vi "Measurement.vi"(0 "Position":T7(array[cluster]) {"Z" format="%.1f"; "Y" format="%.1f"; "X" format="%.1f"}, 1 "setup":T8=enum."Show Setup", 2 "Post Process":T5, 4 "File":T9, 5 "Results file":path, 7 "Raw data file":path, 11 "Setup filename":string) -> (14 "2nd plot":cluster{"Xo":dbl, "Delta X":dbl, dbl[]}[](graph), 19 "Status Out":T4)   [LabVIEW 2011]
uses:
  Anemometry Sub Vis/Controls/Save_Data.ctl
  Anemometry Sub Vis/Controls/Setup.ctl
  Anemometry Sub Vis/Controls/Graph_Type.ctl
  Anemometry Sub Vis/Controls/Post_Process.ctl
  Anemometry Sub Vis/Gen Trav/Multi_Run_Status.ctl
  Anemometry Sub Vis/Controls/Board_Types.ctl
  Anemometry Sub Vis/File/Setup_Filetype.ctl
  Anemometry Sub Vis/Controls/Block_start_and_end.ctl
  ADAM Client/Sub VIs/ADAM Controls/Traverse_Level_State.ctl
  Anemometry Sub Vis/Globals/Trav_pos_global.vi
  Anemometry Sub Vis/Globals/Meas_global.vi
  Anemometry Sub Vis/Acquisition/Data_Translation/DataTranslation_global.vi
  Anemometry Sub Vis/Acquisition/PWA/PWAtasksGLOBAL.vi
  Anemometry Sub Vis/Globals/Preference_global.vi
  Anemometry Sub Vis/Globals/LDA_meas_global_2.vi
  Anemometry Sub Vis/Globals/LDA_meas_global_1.vi
  Anemometry Sub Vis/Globals/Dynamic_call_global.ph.vi
  Anemometry Sub Vis/Globals/Plug_in_data_global.vi
panel:
  in  "PP next block":bool
  out "Pause message":string
  out "Statistics":string[][](table)
  in  "Tab Control":T1(tab)
  out "Measurement time (min)":dbl=6.0 format="%.2f"
  in  "No of bins":i32=80
  in  "Show Smoth":bool=TRUE
  in  "Second Graph":T3={"Plot 1"=2, "Plot 2"=1, "Save graph"=0, "Plot Type"=enum."Vel histogram"} {"Save graph" items=["Do not save plot", "Save plot"]; "Plot 2" items=["Nothing", "LDA (U1)", "LDA (U2)", "HW (Uhw) LDA Sync", "HW (Uhw)", "RV (Sync)"]; "Plot 1" items=["Nothing", "LDA (U1)", "LDA (U2)", "HW (Uhw) LDA Sync", "HW (Uhw)", "RV (Sync)"]}
  in  "First Graph":T3={"Plot 1"=1, "Plot 2"=2, "Save graph"=0, "Plot Type"=enum."Velocity trace"} {"Save graph" items=["Do not save plot", "Save plot"]; "Plot 2" items=["Nothing", "LDA (U1)", "LDA (U2)", "HW (Uhw) LDA Sync", "HW (Uhw)", "RV (Sync)"]; "Plot 1" items=["Nothing", "LDA (U1)", "LDA (U2)", "HW (Uhw) LDA Sync", "HW (Uhw)", "RV (Sync)"]}
  out "First plot":cluster{"Xo":dbl, "Delta X":dbl, dbl[]}[](graph)
  in  "Comments":string
  out "BSA Diagnostic info":string[][](table)
  out "uv":dbl[][](graph)=[[-0.041806189081711534, -0.046435429052714985, -0.04035660097427599, -0.042187605126076694, -0.042052555599004206]]
  out "u^4":dbl[][](graph)
  out "u^3":dbl[][](graph)
  out "u^2":dbl[][](graph)=[[0.09743628875280319, 0.10575821456272283, 0.10126262927293661, 0.09890442087602569, 0.1022948212436432]]
  out "U":dbl[][](graph)=[[0.8295029456391334, 0.8915896983798417, 0.8415763502225625, 0.8394746126219594, 0.8466062785395404]]
  in  "Block average display control":cluster{"Name":string, "Include":bool}[](array[cluster])=[{"Name"="FF (C)", "Include"=FALSE}]
  out "Array U":dbl[][](array[numeric]) format="%.2e"
  out "Array u^2":dbl[][](array[numeric]) format="%.2e"
  out "Actual Sampling freq":dbl=100.0 format="%.1f"
  in  "Desired Sampling freq (Hz)":dbl=100.0 format="%.1f"
  in  "Correlate?":T6(ring)
  out "Current Block No":i32=5
  in  "Pause":bool
  in  "No of Blocks":i32=5
  in  "stop":bool
  in  "No of samples":i32=1000 min=0 step=1
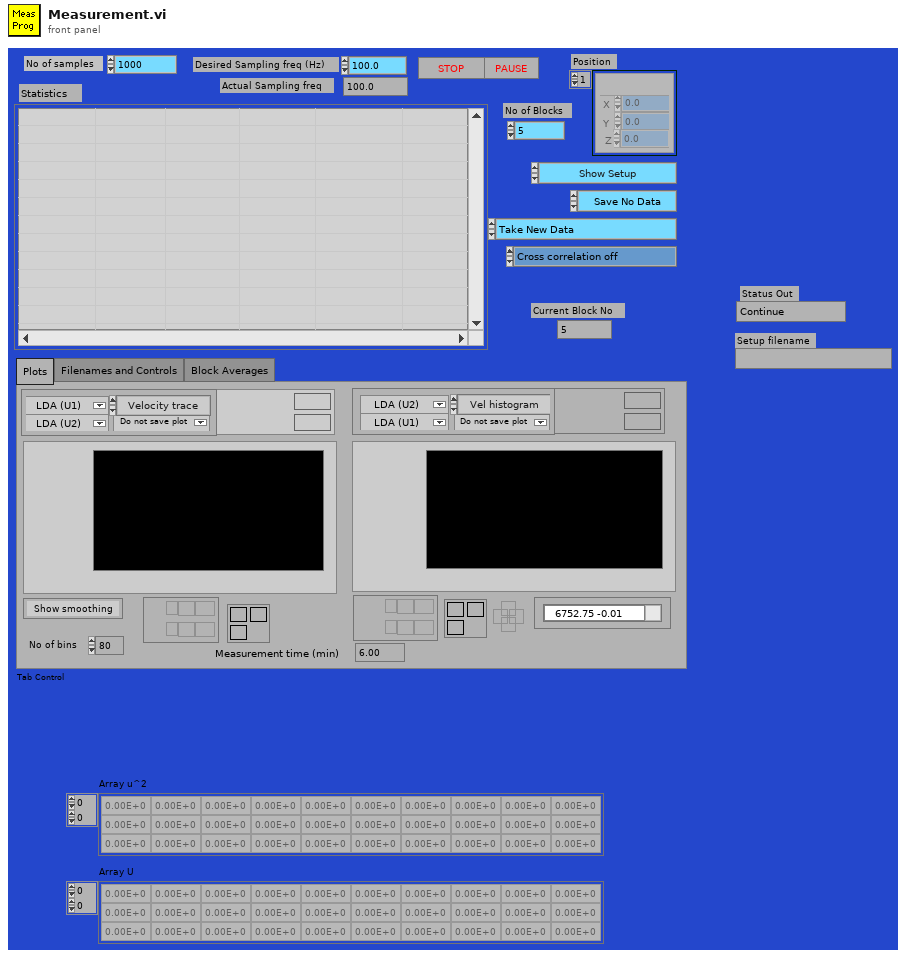
[diagram p1: front panel]
types:
  T1 = enum32{"Plots", "Filenames and Controls", "Block Averages"}
  T2 = typedef "Graph_Type.ctl" = enum16{"Show no graph", "Voltage trace", "Velocity trace", "Vel histogram", "Spectrum", "f.E(f) v Log f", "Auto-Corr"}
  T3 = cluster{"Plot 1":u16, "Plot 2":u16, "Save graph":u16, "Plot Type":T2}
  T4 = typedef "Multi_Run_Status.ctl" = enum16{"Continue", "Jump to Next Point", "Jump to Next Row", "Jump To Fall Back", "Terminate Run"}
  T5 = typedef "Post_Process.ctl" = enum16{"Take New Data", "Post Process Raw Data File"}
  T6 = enum16{"Cross correlation off", "Show correlation panel", "Correlate without activating panel"}
  T7 = cluster{"Name":string, "X":dbl, "Y":dbl, "Z":dbl}[]
  T8 = typedef "Setup.ctl" = enum16{"Run Program", "Show Setup", "Save Current Setup", "Setup Front Panel"}
  T9 = typedef "Save_Data.ctl" = enum16{"Save No Data", "Save Data"}
  T10 = enum32{"Bad", "Idle", "Run top level", "Running"}
  T11 = enum16{"Velocity", "Transit time", "Arrival time"}
  T12 = enum16{"Save no data", "Save data in new files", "Save data in existing files"}
  T13 = typedef "Board_Types.ctl" = enum16{"Simulate", "Local ADAM", "Server ADAM", "NI-DAQmx", "NI-DAQmxBase", "ADC488", "DT LV-link"}
  T14 = typedef "Setup_Filetype.ctl" = enum16{"Measurement Setups", "Calibration Setups", "General", "Results File Plotter Setups", "Speed Calib Tweaks"}
  T15 = typedef "Block_start_and_end.ctl" = cluster{"Started":dbl, "Ended":dbl, "Analogue Frequency Hz":dbl}
  T16 = typedef "Traverse_Level_State.ctl" = enum16{"Running", "Complete"}
  T17 = typedef "Traverse_cluster.ctl" = cluster{"Start X":dbl, "Start Y":dbl, "Start Z":dbl, "End X":dbl, "End Y":dbl, "End Z":dbl, "No. of pts.":i32, "Spacing":T18, "Filename":path, "Tunnel Speed":dbl, "Averaging time (min)":dbl, "Extra Commands":string, "Specific Arguments":string, "Emission Rate (l/min)":dbl, "Trace Gas Concentration (%)":dbl, "Density Ratio":string, "Comments":string, "Row No":i32, "Row Type Selector":T19, "Completion time":string, "Row Duration (mins)":dbl, "No. of Valid pts.":i32, "Meas Setup File":string}
  T18 = typedef "Spacing.ctl" = enum16{"Linear", "Log", "Gauss", "Specified", "N/A"}
  T19 = typedef "Multi_run_mode.ctl" = enum16{"Move Traverse Only", "Set Tunnel Speed Only", "Set Source Only", "Set Measurement Conditions", "Single Measurement", "Vertical Profile", "Lateral Profile", "Longitudinal Profile", "Explore Volume", "Multi-Axis Profile", "Auto Calibrate", "Meas Fast FID Bkgnd", "Check Beam Power", "Scanning Valve Measurement", "Run VI Named:", "Set ADAM Ch", "Wait (minutes)", "Send Message", "Synchronize With:", "Fall Back to this Row", "Turn Off Row Repeating", "Blank Row", "Traverse 3D Volume"}
  T20 = typedef "Analysis_info_cluster.ctl" = cluster{"Colour":u32, "Inst type":T21, "Inst name":string, "Symbol":string, "Code name":string, "Extra Info":string, "Inst Array":T22, "Index":i32, "Voltage Index":i32, "Extra Titles":string[], "Extra Values":string[], "Eng Values":dbl[], "Time (ms)":dbl[], "TT / Voltage":dbl[], "u^2":dbl, "U":dbl, "u^3/(u^2)^(1.5)":dbl, "u^4":dbl, "u^4/(u^2)^2 -3":dbl, "Mean % Err":dbl, "% u'/U":dbl}
  T21 = typedef "Inst_type.ctl" = enum16{"Propeller anemometer", "Raw voltage", "Pressure Transducer", "Pitot-static tube", "Preston tube", "Hot wire", "Cross wire 1", "Cross wire 2", "Generic Linear", "Generic Polynomial", "Generic BackPoly", "Fast FID", "Thermocouple", "Cold wire", "Pulsed Wire", "LDA Vel", "LDA Tran time", "LDA Arr time"}
  T22 = typedef "Instrument_Array.ctl" = enum16{"PWA", "LDA", "Analogue"}
  T23 = enum16{"Velocity", "Transit time", "Arrival time"}[]
  T24 = typedef "BSA_Type.ctl" = enum16{"57N11", "BSA F60"}
  T25 = typedef "BSA_info_Cluster.ctl" = cluster{"GPIB Address":string, "No of Check Bytes":i32, "Extra Info":string, "COLOUR":u32, "Wavelength (nm)":dbl}
  T26 = typedef "Ch_and_Spans.ctl" = cluster{"high limit (10V)":sgl, "low limit (-10V)":sgl, "Ch No":i16, "Var name":string, "Use Latest Calib":bool}
  T27 = typedef "Velocity_cluster.ctl" = cluster{"Name":string, "U":dbl, "u^2":dbl, "u^3/(u^2)^(1.5)":dbl, "u^4/(u^2)^2 -3":dbl, "% u'/U":dbl, "Mean % Err":dbl, "u^4":dbl}
  T28 = typedef "Analysis_type_cluster.ctl" = cluster{"Analysis type":T29, "Indicies":i32[], "Name":string, "Inst Array":T22, "Info index":i32}
  T29 = typedef "Analysis_type_Enum.ctl" = enum16{"Slow Response", "Fast Response", "Weighted Fast Response", "Fast FID", "Weighted Fast FID", "Cross Wire", "Weighted Cross Wire", "Weighted LDA"}
  T30 = cluster{"Insts for plotting[0]":u16, "Insts for plotting[1]":u16}
  T31 = typedef "PWA_Data.ctl" = enum16{"No PWA Data", "One Ch PWA"}
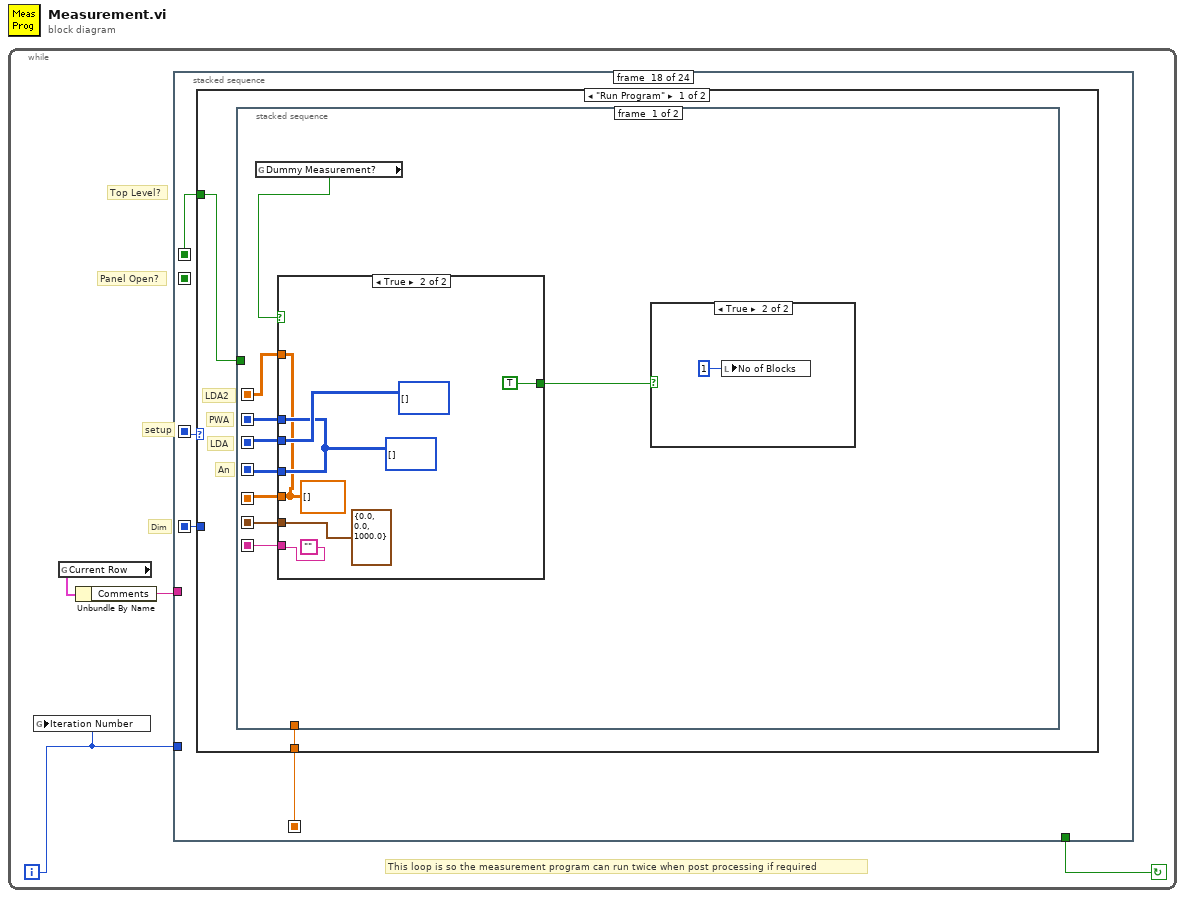
[diagram p0: block diagram]
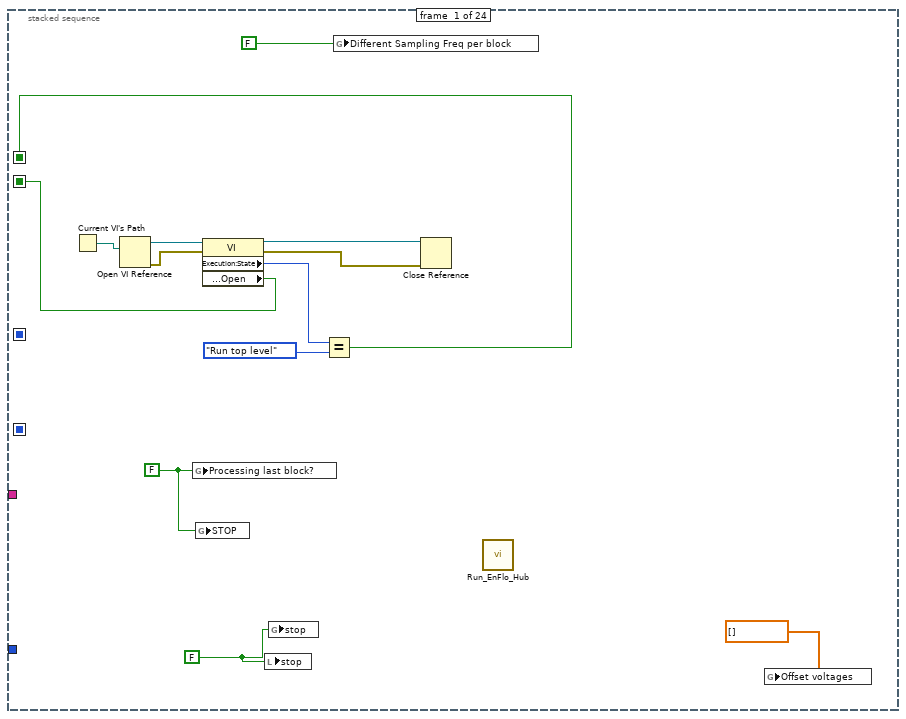
[diagram p2: hidden frame]
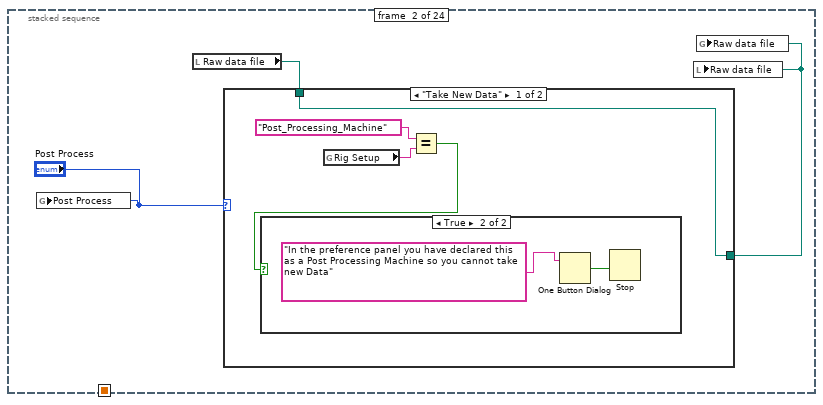
[diagram p3: hidden frame]
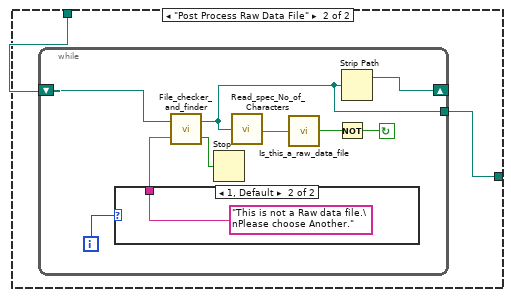
[diagram p5: hidden frame]
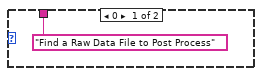
[diagram p6: hidden frame]
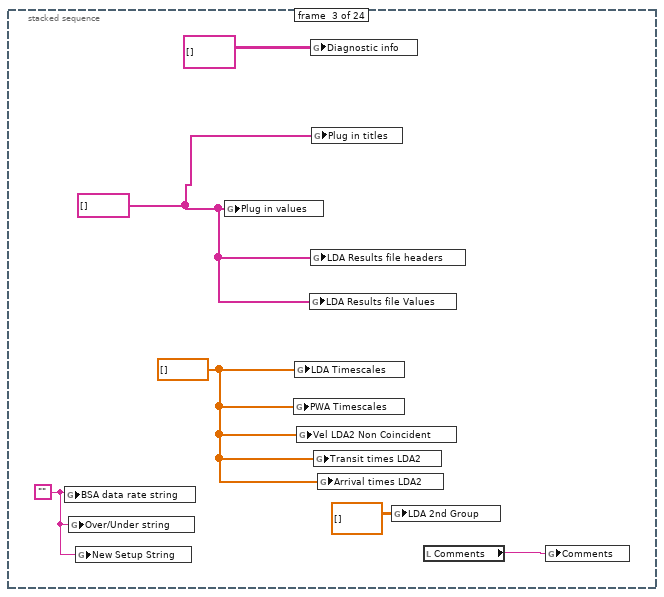
[diagram p7: hidden frame]
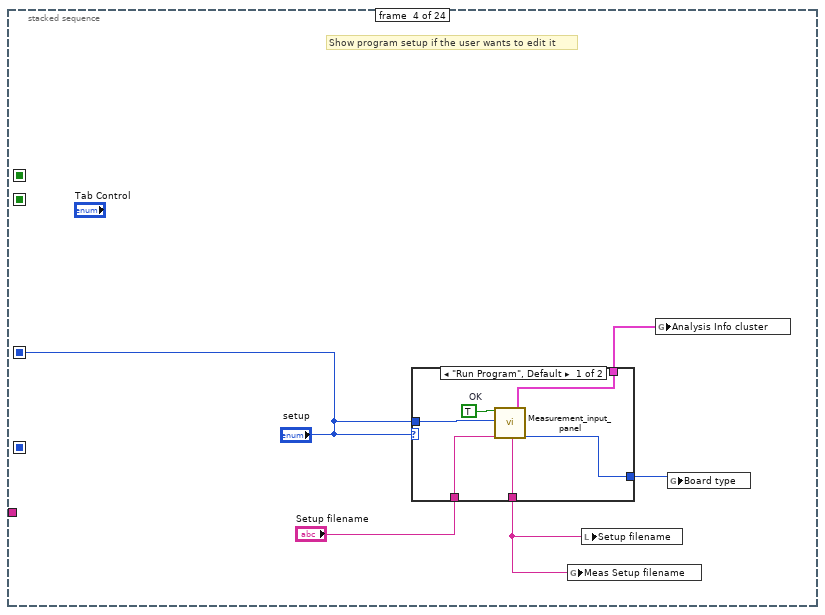
[diagram p8: hidden frame]
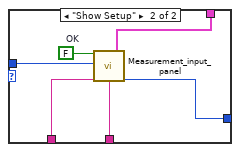
[diagram p9: hidden frame]
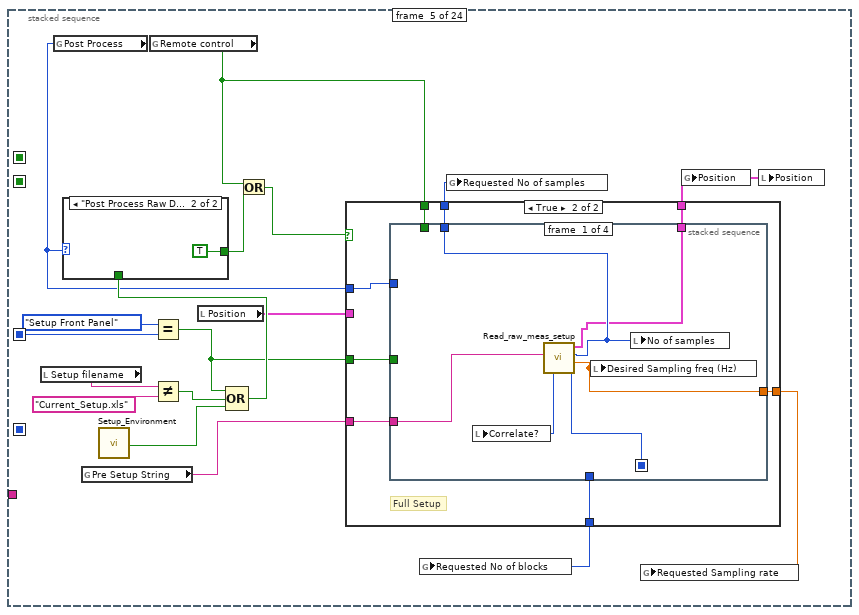
[diagram p10: hidden frame]
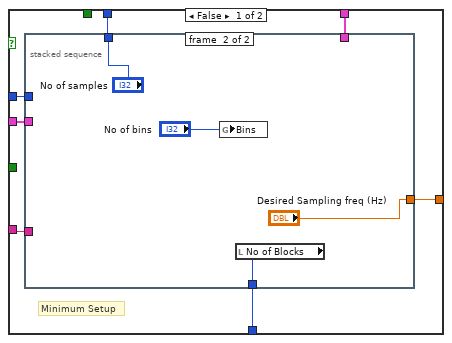
[diagram p12: hidden frame]
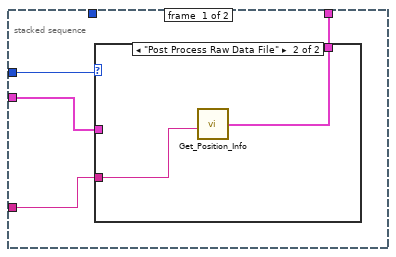
[diagram p13: hidden frame]
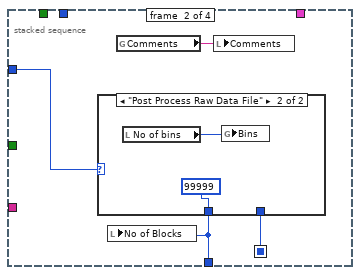
[diagram p15: hidden frame]
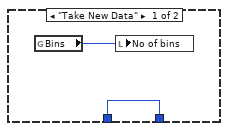
[diagram p16: hidden frame]
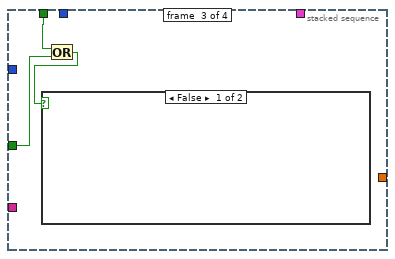
[diagram p17: hidden frame]
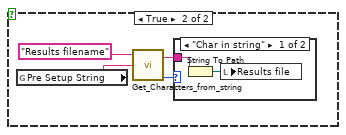
[diagram p18: hidden frame]
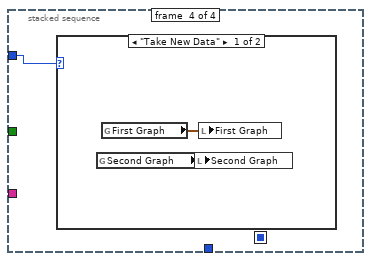
[diagram p20: hidden frame]
diagram:
  n1 = while {
    i -> [w1]
    stop <- w2 continue-if-true
    # "This loop is so the measurement program can run twice when post processing if required"
    # "Panel Open?"
    # "Top Level?"
    # "setup"
    # "Dim"
    n2 = global write "Meas_global.vi" "Iteration Number"(w1) -> ()
    n3 = global read "Trav_pos_global.vi" "Current Row"() -> (w3:T17)
    n4 = Unbundle By Name(w3) -> ("Comments"=w4:string)
    n5 = stacked-sequence {
      seq-local: [_ _ _ _ _ _ _ _ w188 _ _ _ _ _ _ _ _ _ _ _ _ _ _ _] -> [_ _ _ _ _ _ _ _ _ _ _ _ _ _ _ _ _ w627 _ _ _ _ _ _]
      seq-local: [_ _ _ "setup" _ _ _ _ _ _ _ _ _ _ _ _ _ _ _ _ _ _ _ _] -> [_ _ _ _ w72 _ _ _ w180 w265 _ _ _ _ w525 w565 w572 w628 w944 w1020 w1046 _ _ w1121]
      seq-local: [_ _ _ _ _ _ _ _ _ _ _ _ _ _ _ _ w568 _ _ _ _ _ _ _] -> [_ _ _ _ _ _ _ _ _ _ _ _ _ _ _ _ _ w626 w927 _ _ _ _ _]
      seq-local: [w7 _ _ _ _ _ _ _ _ _ _ _ _ _ _ _ _ _ _ _ _ _ _ _] -> [_ _ _ _ _ _ _ _ _ w245 _ _ _ _ w521 _ _ w625 _ _ _ _ _ _]
      seq-local: [w6 _ _ _ _ _ _ _ _ _ _ _ _ _ _ _ _ _ _ _ _ _ _ _] -> [_ _ _ _ _ _ _ _ _ _ _ _ w364 _ _ _ _ _ _ _ _ _ _ _]
      tunnel: w4 -> [_ _ _ _ _ _ _ w173 _ _ _ _ _ _ _ _ _ _ _ _ _ _ w1089 _]
      tunnel: w1 -> [_ _ _ _ _ _ _ _ _ _ _ _ _ _ _ _ _ _ _ _ _ _ w1084 _]
      tunnel: [_ _ _ _ _ _ _ _ _ _ _ _ _ _ _ _ _ _ _ _ _ _ w1083 _] -> w2
      frame #0 {
        w15 = FALSE ("Processing last block?")
        w16 = FALSE ("stop")
        n6 = Current VI's Path() -> (path=w8:path)
        n7 = Open VI Reference(vi path=w8) -> (vi reference=w9:refnum<vi>, error out=w10:errorcluster)  [unwired: 1 in, 4 out]
        n8 = global write "Meas_global.vi" "Processing last block?"(w15) -> ()
        n9 = global write "PWAtasksGLOBAL.vi" "STOP"(w15) -> ()
        n10 = property class="VI"(reference=w9, error in=w10) -> (reference out=w11:refnum<vi>, error out=w12:errorcluster, "Execution:State"=w13:T10, "Front Panel.Open"=w6:bool)
        n11 = local write "stop"(w16) -> ()
        n12 = global write "Meas_global.vi" "stop"(w16) -> ()
        n13 = Equal?(x=w13, y=T10."Run top level" ("Exec.State")) -> (x = y?=w7:bool)
        n14 = global write "DataTranslation_global.vi" "Different Sampling Freq per block"(FALSE ("Different Sampling Freq per block")) -> ()
        n15 = Close Reference(reference=w11, error in (no error)=w12) -> ()  [unwired: 1 out]
        n16 = call "Run_EnFlo_Hub.vi"() -> ()  [unwired: 8 out]
        n17 = global write "Meas_global.vi" "Offset voltages"(dbl[] [] ("Offset voltages used")) -> ()
      }
      frame #1 {
        n18 = global write "Meas_global.vi" "Post Process"("Post Process") -> ()
        n19 = local read "Raw data file"() -> (w20:path)
        n20 = case shown="\"Take New Data\"" "Post Process" {
          tunnel: [w24 w28] -> w19
          tunnel: w20 -> [w24 w27]
          frame "Take New Data" {
            n21 = global read "Preference_global.vi" "Rig Setup"() -> (w23:string)
            n22 = Equal?(x="Post_Processing_Machine" ("Rig Setup"), y=w23) -> (x = y?=w21:bool)
            n23 = case shown="True" w21 {
              frame False {
              }
              frame True {
                n24 = One Button Dialog(message="In the preference panel you have declared this as a Post Processing Machine so you cannot take new Data") -> (true=w25:bool)  [unwired: 1 in]
                n25 = Stop(stop? (T)=w25) -> ()
              }
            }
          }
          frame "Post Process Raw Data File" {
            n26 = while {
              tunnel: [w30] -> w28
              shift-left: w27 -> [w32]
              shift-right: [w31] -> _
              i -> [w33]
              stop <- w34 continue-if-true
              n27 = case shown="1, Default" w33 {
                tunnel: ["Find a Raw Data File to Post Process" ("Promp if not found") "This is not a Raw data file.\nPlease choose Another." ("Promp if not found")] -> w37
                frame 0 {
                }
                frame 1, Default {
                }
              }
              n28 = call "File_checker_and_finder.vi"("Promp if not found"=w37, "Filename In"=w32) -> ("cancelled"=w29:bool, "Filename Out"=w30:path)
              n29 = Stop(stop? (T)=w29) -> ()
              n30 = call "Read_spec_No_of_Characters.vi"("Filename"=w30) -> ("character string"=w36:string)  [unwired: 1 out]
              n31 = call "Is_this_a_raw_data_file.vi"("character string"=w36) -> ("Raw Dat File?"=w35:bool)  [unwired: 2 out]
              n32 = Not(x=w35) -> (.not. x?=w34:bool)
              n33 = Strip Path(path=w30) -> (stripped path=w31:path)  [unwired: 1 out]
            }
          }
        }
        n34 = local write "Raw data file"(w19) -> ()
        n35 = global write "Meas_global.vi" "Raw data file"(w19) -> ()
      }
      frame #2 {
        w40 = dbl[] [] ("LDA Timescales")
        w43 = string[] [] ("Plug in values")
        w45 = ""
        n36 = global write "Meas_global.vi" "BSA data rate string"(w45) -> ()
        n37 = global write "Meas_global.vi" "Over/Under string"(w45) -> ()
        n38 = global write "Meas_global.vi" "New Setup String"(w45) -> ()
        n39 = global write "Dynamic_call_global.ph.vi" "Plug in values"(w43) -> ()
        n40 = global write "PWAtasksGLOBAL.vi" "PWA Timescales"(w40) -> ()
        n41 = global write "LDA_meas_global_1.vi" "LDA Timescales"(w40) -> ()
        n42 = global write "LDA_meas_global_2.vi" "Vel LDA2 Non Coincident"(w40) -> ()
        n43 = global write "LDA_meas_global_1.vi" "LDA Results file Values"(w43) -> ()
        n44 = global write "Meas_global.vi" "Diagnostic info"(string[][] [] ("Diagnostic info")) -> ()
        n45 = global write "LDA_meas_global_1.vi" "LDA Results file headers"(w43) -> ()
        n46 = global write "Dynamic_call_global.ph.vi" "Plug in titles"(w43) -> ()
        n47 = global write "LDA_meas_global_2.vi" "Transit times LDA2"(w40) -> ()
        n48 = global write "LDA_meas_global_2.vi" "Arrival times LDA2"(w40) -> ()
        n49 = global write "LDA_meas_global_2.vi" "LDA 2nd Group"(dbl[][] [] ("LDA 2nd Group")) -> ()
        n50 = local read "Comments"() -> (w44:string)
        n51 = global write "Meas_global.vi" "Comments"(w44) -> ()
      }
      frame #3 {
        # "Show program setup if the user wants to edit it"
        n52 = case shown="\"Run Program\", Default" "setup" {
          tunnel: [w55 w61] -> w50
          tunnel: [w54 w60] -> w49
          tunnel: "Setup filename" -> [w53 w59]
          tunnel: [w52 w58] -> w46
          tunnel: "setup" -> [w51 w57]
          frame "Run Program", Default {
            w56 = TRUE  # OK
            n53 = call "Measurement_input_panel.vi"("OK"=w56, "setup"=w51, "Setup filename"=w53) -> ("Setup filename out"=w52:string, "Analysis Info cluster"=w55:T20[], "Board type"=w54:T13)  [unwired: 14 out]
          }
          frame "Show Setup" {
            w62 = FALSE  # OK
            n54 = call "Measurement_input_panel.vi"("OK"=w62, "setup"=w57, "Setup filename"=w59) -> ("Setup filename out"=w58:string, "Analysis Info cluster"=w61:T20[], "Board type"=w60:T13)  [unwired: 14 out]
          }
        }
        n55 = global write "Meas_global.vi" "Meas Setup filename"(w46) -> ()
        n56 = local write "Setup filename"(w46) -> ()
        n57 = global write "Meas_global.vi" "Analysis Info cluster"(w50) -> ()
        n58 = global write "Meas_global.vi" "Board type"(w49) -> ()
      }
      frame #4 {
        n59 = local read "Setup filename"() -> (w76:string)
        n60 = global read "Meas_global.vi" "Post Process"() -> (w71:T5)
        n61 = global read "Meas_global.vi" "Pre Setup String"() -> (w67:string)
        n62 = call "Setup_Environment.vi"() -> ("First Time"=w68:bool)  [unwired: 1 in]
        n63 = global read "Meas_global.vi" "Remote control"() -> (w64:bool)
        n64 = Equal?(x=Setup."Setup Front Panel" ("setup"), y=w72) -> (x = y?=w63:bool)
        n65 = Not Equal?(x=w76, y="Current_Setup.xls" ("Setup filename")) -> (x != y?=w74:bool)
        n66 = local read "Position"() -> (w65:T7)
        n67 = Compound Arithmetic op=OR(w63, w74, w68) -> (w73:bool)
        n68 = case shown="\"Post Process Raw Data File\"" w71 {
          tunnel: [w81 TRUE] -> w80
          tunnel: w73 -> [w81 _]
          frame "Take New Data" {
          }
          frame "Post Process Raw Data File" {
          }
        }
        n69 = Or(x=w64, y=w80) -> (x .or. y?=w79:bool)
        n70 = case shown="True" w79 {
          tunnel: w71 -> [w85 w108]
          tunnel: [w89 w107] -> w69
          tunnel: [w88 w102] -> w78
          tunnel: [w87 w106] -> w77
          tunnel: [w86 w105] -> w66
          tunnel: w67 -> [w84 w104]
          tunnel: w65 -> [w83 _]
          tunnel: w64 -> [_ w103]
          tunnel: w63 -> [_ w101]
          frame False {
            # "Minimum Setup"
            n71 = stacked-sequence {
              tunnel: [_ "Desired Sampling freq (Hz)"] -> w89
              tunnel: [_ w99] -> w88
              tunnel: [_ "No of samples"] -> w87
              tunnel: [w92 _] -> w86
              tunnel: w85 -> [w93 _]
              tunnel: w84 -> [w91 _]
              tunnel: w83 -> [w90 _]
              frame #0 {
                n72 = case shown="\"Post Process Raw Data File\"" w93 {
                  tunnel: [w94 w95] -> w92
                  tunnel: w90 -> [w94 _]
                  tunnel: w91 -> [_ w96]
                  frame "Take New Data" {
                  }
                  frame "Post Process Raw Data File" {
                    n73 = call "Get_Position_Info.vi"("Input string"=w96) -> ("Position"=w95:T7)
                  }
                }
              }
              frame #1 {
                n74 = global write "Meas_global.vi" "Bins"("No of bins") -> ()
                n75 = local read "No of Blocks"() -> (w99:i32)
              }
            }
          }
          frame True {
            # "Full Setup"
            n76 = stacked-sequence {
              seq-local: [w111 _ _ _] -> [_ w116 _ _]
              tunnel: w108 -> [_ w117 _ w132]
              tunnel: [w114 _ _ _] -> w107
              tunnel: [w113 _ _ _] -> w106
              tunnel: [w109 _ _ _] -> w105
              tunnel: w104 -> [w112 _ _ _]
              tunnel: w103 -> [_ _ w125 _]
              tunnel: [_ w115 _ _] -> w102
              tunnel: w101 -> [_ _ w124 _]
              frame #0 {
                n77 = call "Read_raw_meas_setup.vi"("Setup file string"=w112) -> ("No of Blocks"=w111:i32, "Sampling freq (Hz)"=w114:dbl, "No of samples"=w113:i32, "Position"=w109:T7, "Correlate?"=w110:T6)  [unwired: 4 out]
                n78 = local write "Correlate?"(w110) -> ()
                n79 = local write "Desired Sampling freq (Hz)"(w114) -> ()
                n80 = local write "No of samples"(w113) -> ()
              }
              frame #1 {
                n81 = case shown="\"Post Process Raw Data File\"" w117 {
                  tunnel: [w120 99999 ("No of Blocks")] -> w115
                  tunnel: w116 -> [w120 _]
                  frame "Take New Data" {
                    n82 = global read "Meas_global.vi" "Bins"() -> (w119:i32)
                    n83 = local write "No of bins"(w119) -> ()
                  }
                  frame "Post Process Raw Data File" {
                    n84 = local read "No of bins"() -> (w121:i32)
                    n85 = global write "Meas_global.vi" "Bins"(w121) -> ()
                  }
                }
                n86 = local write "No of Blocks"(w115) -> ()
                n87 = global read "Meas_global.vi" "Comments"() -> (w118:string)
                n88 = local write "Comments"(w118) -> ()
              }
              frame #2 {
                n89 = Or(x=w125, y=w124) -> (x .or. y?=w123:bool)
                n90 = case shown="False" w123 {
                  frame False {
                  }
                  frame True {
                    n91 = global read "Meas_global.vi" "Pre Setup String"() -> (w126:string)
                    n92 = call "Get_Characters_from_string.vi"("Input string"=w126, "Variable name"="Results filename") -> ("Status"=w129:enum16{"Char in string", "Char not in string"}, "Value"=w128:string)  [unwired: 1 in]
                    n93 = case shown="\"Char in string\"" w129 {
                      tunnel: w128 -> [w131 _]
                      frame "Char in string" {
                        n94 = String To Path(string=w131) -> (path=w130:path)
                        n95 = local write "Results file"(w130) -> ()
                      }
                      frame "Char not in string" {
                      }
                    }
                  }
                }
              }
              frame #3 {
                n96 = case shown="\"Take New Data\"" w132 {
                  frame "Take New Data" {
                    n97 = global read "Meas_global.vi" "Second Graph"() -> (w133:T3)
                    n98 = global read "Meas_global.vi" "First Graph"() -> (w134:T3)
                    n99 = local write "Second Graph"(w133) -> ()
                    n100 = local write "First Graph"(w134) -> ()
                  }
                  frame "Post Process Raw Data File" {
                  }
                }
              }
            }
          }
        }
        n101 = global write "Meas_global.vi" "Requested No of blocks"(w78) -> ()
        n102 = global write "Meas_global.vi" "Requested No of samples"(w77) -> ()
        n103 = global write "Meas_global.vi" "Requested Sampling rate"(w69) -> ()
        n104 = global write "Meas_global.vi" "Position"(w66) -> ()
        n105 = local write "Position"(w66) -> ()
      }
      frame #5 {
        n106 = global read "Meas_global.vi" "Post Process"() -> (w135:T5)
        n107 = case shown="\"Post Process Raw Data File\"" w135 {
          tunnel: [w138 w139] -> w136
          frame "Take New Data" {
            n108 = Get Date/Time In Seconds() -> (seconds since 1Jan1904=w137:timestamp)
            n109 = To Double Precision Float(number=w137) -> (double precision float=w138:dbl)
          }
          frame "Post Process Raw Data File" {
            n110 = global read "Meas_global.vi" "Pre Setup String"() -> (w142:string)
            n111 = call "Get_Characters_from_string.vi"("Input string"=w142, "Variable name"="Seconds since 1/1/04") -> ("Value"=w140:string)  [unwired: 1 in, 1 out]
            n112 = call "String_2_Number.vi"("Value"=w140) -> ("Numeric"=w139:dbl)
          }
        }
        n113 = global write "Meas_global.vi" "Time Data was Aquired"(w136) -> ()
      }
      frame #6 {
        n114 = global read "Dynamic_call_global.ph.vi" "Initial Plug Ins"() -> (w144:string[])
        n115 = global read "Dynamic_call_global.ph.vi" "Initial Plug Ins Extra"() -> (w145:string[])
        n116 = Build Array (concatenate)(w145, w144) -> (w143:string[])
        n117 = Array Size(array=w143) -> (size(s)=w147:i32)
        n118 = Greater Than 0?(x=w147) -> (x > 0?=w146:bool)
        n119 = case shown="True" w146 {
          tunnel: w143 -> [_ w148]
          frame False {
          }
          frame True {
            n120 = stacked-sequence {
              tunnel: w148 -> [w150 _]
              frame #0 {
                n121 = global read "Meas_global.vi" "Post Process"() -> (w152:T5)
                n122 = call "Plug_in_Directories.vi"() -> ("Initial"=w149:path)  [unwired: 3 out]
                n123 = Equal?(x=w152, y=Post_Process."Post Process Raw Data File" ("Post Process")) -> (x = y?=w151:bool)
                n124 = for {
                  tunnel: w151 -> [w158]
                  tunnel: w150 -> [w155] mode=indexing
                  tunnel: w149 -> [w154]
                  w165 = FALSE  # Dialog Box (T)
                  n125 = Build Path(base path=w154, name or relative path=w155) -> (appended path=w156:path)
                  n126 = Open VI Reference(vi path=w156) -> (vi reference=w163:refnum<vi>, error out=w162:errorcluster)  [unwired: 2 in, 3 out]
                  n127 = property class="VI"(reference=w163, error in=w162, "Front Panel Window:Open"=TRUE ("Wait until done")) -> (reference out=w161:refnum<vi>, error out=w160:errorcluster)
                  n128 = invoke class="VI" method="Run VI"(reference=w161, error in=w160, "Wait until done"=w158, "Auto Dispose Ref"=FALSE) -> (reference out=w168:refnum<vi>, error out=w167:errorcluster)  [unwired: 1 in, 3 out]
                  n129 = Close Reference(reference=w168, error in (no error)=w167) -> (error out=w166:errorcluster)
                  n130 = call "EnFlo_Error_Handler.vi"("error in (no error)"=w166, "Error Type"="Launching Initial Plug In", "Dialog Box (T)"=w165) -> ()  [unwired: 3 out]
                }
              }
              frame #1 {
                n131 = global read "Meas_global.vi" "Requested No of blocks"() -> (w170:i32)
                n132 = global read "Meas_global.vi" "Comments"() -> (w169:string)
                n133 = local write "Comments"(w169) -> ()
                n134 = local write "No of Blocks"(w170) -> ()
              }
            }
          }
        }
      }
      frame #7 {
        n135 = local read "Comments"() -> (w174:string)
        n136 = Concatenate Strings(w173, w174) -> (w172:string)
        n137 = call "Text_without_format.vi"("Input string"=w172) -> ("Output string"=w171:string)
        n138 = local write "Comments"(w171) -> ()
        n139 = global write "Meas_global.vi" "Comments"(w171) -> ()
      }
      frame #8 {
        n140 = global read "Meas_global.vi" "dimensions"() -> (w188:enum16{"1D", "2D"})
        n141 = global read "Meas_global.vi" "Post Process"() -> (w187:T5)
        n142 = global read "Meas_global.vi" "LDA data"() -> (w185:enum16{"No LDA data", "Take LDA data"})
        n143 = Equal?(x=Setup."Run Program" ("setup"), y=w180) -> (x = y?=w183:bool)
        n144 = Equal?(x=w180, y=Setup."Show Setup" ("setup")) -> (x = y?=w175:bool)
        n145 = Equal?(x=w185, y=enum16{"No LDA data", "Take LDA data"}."Take LDA data" ("LDA data")) -> (x = y?=w178:bool)
        n146 = Or(x=w183, y=w175) -> (x .or. y?=w177:bool)
        n147 = Equal?(x=w187, y=Post_Process."Take New Data" ("Post Process")) -> (x = y?=w179:bool)
        n148 = Compound Arithmetic op=AND(w177, w178, w179) -> (w176:bool)
        n149 = case shown="True" w176 {
          tunnel: w188 -> [_ w197]
          tunnel: w180 -> [_ w196]
          tunnel: w175 -> [_ w194]
          frame False {
            n150 = Build Array(T11."Velocity", T11."Transit time", T11."Arrival time") -> (w189:T23)
            n151 = global write "LDA_meas_global_1.vi" "Number of measured quantities"(3 ("Number of measured quantities")) -> ()
            n152 = global write "LDA_meas_global_2.vi" "data type"(w189) -> ()
            n153 = global write "LDA_meas_global_1.vi" "data type"(w189) -> ()
          }
          frame True {
            n154 = global read "LDA_meas_global_1.vi" "BSA Type"() -> (w195:T24)
            n155 = case shown="\"BSA F60\"" w195 {
              tunnel: w197 -> [w199 _]
              tunnel: w196 -> [w198 _]
              tunnel: w194 -> [_ w235]
              frame "57N11" {
                n156 = stacked-sequence {
                  tunnel: w199 -> [w202 w228]
                  tunnel: w198 -> [w201 _]
                  frame #0 {
                    n157 = global read "Meas_global.vi" "Remote control"() -> (w200:bool)
                    n158 = case shown="\"2D\"" w202 {
                      tunnel: w201 -> [w204 w217]
                      tunnel: w200 -> [w203 w216]
                      frame "2D" {
                        n159 = while {
                          tunnel: w203 -> [w205]
                          tunnel: w204 -> [w206]
                          stop <- w207 continue-if-true
                          n160 = stacked-sequence {
                            tunnel: [_ _ w213] -> w207
                            tunnel: w206 -> [w208 w210 _]
                            tunnel: w205 -> [_ _ w212]
                            frame #0 {
                              w209 = "1"  # BSA Number
                              n161 = call "Control_BSA_setup.vi"("setup"=w208, "BSA number"=w209) -> ()  [unwired: 14 out]
                            }
                            frame #1 {
                              w211 = "2"  # BSA Number
                              n162 = call "Control_BSA_setup.vi"("setup"=w210, "BSA number"=w211) -> ()  [unwired: 14 out]
                            }
                            frame #2 {
                              n163 = case shown="False" w212 {
                                tunnel: [w214 FALSE ("ok")] -> w213
                                frame False {
                                n164 = call "BSA_setup_check.vi"() -> ("ok"=w214:bool)
                                }
                                frame True {
                                }
                              }
                            }
                          }
                        }
                      }
                      frame "1D" {
                        n165 = stacked-sequence {
                          tunnel: w217 -> [w218 _]
                          tunnel: w216 -> [_ _]
                          frame #0 {
                            w219 = "1"  # BSA Number
                            n166 = call "Control_BSA_setup.vi"("setup"=w218, "BSA number"=w219) -> ()  [unwired: 14 out]
                          }
                          frame #1 {
                            n167 = global read "LDA_meas_global_2.vi" "BSA2 info"() -> (w220:T25)
                            n168 = Unbundle By Name(w220) -> ("GPIB Address"=w221:string)
                            n169 = call "Set_BSA_Coincidence.vi"("GPIB address"=w221, "Set Coincidence"=enum16{"Slave", "Master", "Private"}."Slave") -> ()  [unwired: 1 in, 5 out]
                          }
                        }
                      }
                    }
                  }
                  frame #1 {
                    n170 = global read "Meas_global.vi" "Remote control"() -> (w226:bool)
                    n171 = Equal?(x=w228, y=enum16{"1D", "2D"}."2D" ("dimensions")) -> (x = y?=w224:bool)
                    n172 = Not(x=w226) -> (.not. x?=w225:bool)
                    n173 = And(x=w225, y=w224) -> (x .and. y?=w223:bool)
                    n174 = case shown="True" w223 {
                      frame False {
                      }
                      frame True {
                        n175 = global read "LDA_meas_global_1.vi" "BSA1 info"() -> (w230:T25)
                        n176 = global read "LDA_meas_global_2.vi" "BSA2 info"() -> (w231:T25)
                        n177 = Build Array(w230, w231) -> (w229:T25[])
                        n178 = for {
                          tunnel: w229 -> [w233] mode=indexing
                          n179 = Unbundle By Name(w233) -> ("GPIB Address"=w232:string)
                          n180 = call "Set_BSA_Coincidence.vi"("GPIB address"=w232, "Set Coincidence"=enum16{"Slave", "Master", "Private"}."Master") -> ()  [unwired: 1 in, 5 out]
                        }
                      }
                    }
                  }
                }
              }
              frame "BSA F60" {
                n181 = disable-structure shown="TARGET_TYPE==Windows" {
                  disable-tunnel: w235 -> [_ w236]
                  frame condition #0 (active) {
                  }
                  frame condition #1 {
                    n182 = while {
                      tunnel: w236 -> [w239]
                      stop <- w237 continue-if-true
                      n183 = call "Edit_BSA_IP.vi"("Show Panel"=w239) -> ("Run LDA Diagnostic Out"=w238:bool)  [unwired: 2 out]
                      n184 = case shown="False" w238 {
                        tunnel: [FALSE w241] -> w237
                        frame False {
                        }
                        frame True {
                          n185 = call "F60_Diagnostic.vi"() -> ("Edit BSA Setup Out"=w241:bool)  [unwired: 11 in]
                        }
                      }
                    }
                  }
                }
              }
            }
          }
        }
      }
      frame #9 {
        w250 = Save_Data."Save No Data" ("File")
        w266 = Post_Process."Take New Data"  # Post Process
        n186 = global read "Trav_pos_global.vi" "Meas Setup Number"() -> (w246:i32)
        n187 = Not Equal?(x=Setup."Run Program" ("setup"), y=w265) -> (x != y?=w251:bool)
        n188 = call "Current_Filepath.vi"("Filename in"="Results file", "Data Type"="Results") -> ("Filename Out"=w244:path)  [unwired: 1 out]
        n189 = global read "Meas_global.vi" "Remote control"() -> (w262:bool)
        n190 = global read "Meas_global.vi" "Post Process"() -> (w253:T5)
        n191 = Equal?(x="File", y=w250) -> (x = y?=w260:bool)
        n192 = case shown="1, Default" w246 {
          tunnel: [w269 w271] -> w247
          tunnel: w244 -> [w269 w278]
          tunnel: w246 -> [_ w279]
          frame 0 {
          }
          frame 1, Default {
            n193 = Add(x=96, y=w279) -> (x+y=w281:i32)
            n194 = Build Array(w281) -> (w282:i32[])
            n195 = Strip Path(path=w278) -> (stripped path=w272:path, name=w277:string)
            n196 = Byte Array To String(unsigned byte array=w282) -> (string=w275:string)
            n197 = call "Add_filename_suffix.vi"("Filename"=w277) -> ("Original Suffix"=w274:string, "Base name"=w276:string)  [unwired: 1 in, 2 out]
            n198 = Format Into String(format string="%s_%s%s", w276, w275, w274) -> (resulting string=w273:string)  [unwired: 2 in, 1 out]
            n199 = Build Path(base path=w272, name or relative path=w273) -> (appended path=w271:path)
          }
        }
        n200 = Equal?(x=w253, y=w266) -> (x = y?=w252:bool)
        n201 = And(x=w262, y=w252) -> (x .and. y?=w258:bool)
        n202 = Compound Arithmetic op=AND(w260, invert w262, w252, invert w251) -> (w261:bool)
        n203 = while {
          shift-left: _ -> [w287]
          shift-right: [w284] -> _
          tunnel: "File" -> [w285]
          tunnel: [w288] -> w259
          tunnel: w261 -> [w284]
          stop <- FALSE continue-if-true
          n204 = Compound Arithmetic op=AND(w284, invert w287) -> (w286:bool)
          n205 = case shown="True" w286 {
            tunnel: [w289 w292] -> w288
            tunnel: w285 -> [w289 _]
            frame False {
            }
            frame True {
              n206 = Two Button Dialog(message="Do you wish to save the data?", 1:"Save Data" ("F button name (\"Cancel\")"), 2:"Save No Data" ("T button name (\"OK\")")) -> (T button?=w293:bool)
              n207 = Select(t=Save_Data."Save No Data" ("File"), s=w293, f=Save_Data."Save Data" ("File")) -> (s? t:f=w292:T9)
            }
          }
        }
        n208 = Equal?(x=w250, y=w259) -> (x = y?=w249:bool)
        n209 = Or(x=w249, y=w251) -> (x .or. y?=w264:bool)
        n210 = case shown="False" w264 {
          tunnel: w247 -> [w308 w316]
          tunnel: [w307 w316] -> w267
          tunnel: "Raw data file" -> [w306 w317]
          tunnel: [w301 w317] -> w256
          tunnel: w265 -> [w305 _]
          tunnel: w259 -> [w304 _]
          tunnel: [w302 T12."Save no data" ("File output")] -> w254
          tunnel: [w303 w314] -> w248
          tunnel: w258 -> [_ w311]
          tunnel: w251 -> [_ w310]
          tunnel: w245 -> [w300 _]
          frame False {
            n211 = call "File_setup.vi"("Measurement is top level?"=w300, "Results file"=w308, "Raw data file"=w306, "setup"=w305, "File"=w304) -> ("Results file output"=w307:path, "Raw data file output"=w301:path, "Raw data option"=w303:enum16{"Save raw data", "Raw data not saved"}, "File output"=w302:T12)
          }
          frame True {
            w312 = enum16{"Save raw data", "Raw data not saved"}."Raw data not saved"  # Raw data option
            n212 = global read "Meas_global.vi" "Raw data option"() -> (w313:enum16{"Save raw data", "Raw data not saved"})
            n213 = Compound Arithmetic op=AND(w311, invert w310) -> (w309:bool)
            n214 = Select(t=w313, s=w309, f=w312) -> (s? t:f=w314:enum16{"Save raw data", "Raw data not saved"})
          }
        }
        n215 = case shown="\"Save raw data\"" w248 {
          tunnel: w256 -> [w297 w299]
          tunnel: [w297 w298] -> w255
          frame "Raw data not saved" {
          }
          frame "Save raw data" {
            n216 = call "Find_Unique_Filename.vi"("Path In"=w299) -> ("Unique Path Out"=w298:path)  [unwired: 1 in, 1 out]
          }
        }
        n217 = local write "Results file"(w267) -> ()
        n218 = global write "Meas_global.vi" "Results file"(w267) -> ()
        n219 = global write "Meas_global.vi" "Raw data option"(w248) -> ()
        n220 = global write "Meas_global.vi" "File"(w254) -> ()
        n221 = global write "Meas_global.vi" "Raw data file"(w255) -> ()
        n222 = local write "Raw data file"(w255) -> ()
        n223 = local write "File"(w259) -> ()
      }
      frame #10 {
        n224 = global read "Meas_global.vi" "Ch & spans"() -> (w318:T26[])
        n225 = local read "Block average display control"() -> (w323:cluster{"Name":string, "Include":bool}[])
        n226 = global read "Meas_global.vi" "Velocity Cluster Array"() -> (w322:T27[])
        n227 = global write "Meas_global.vi" "Ch & spans + mod limits"(w318) -> ()
        n228 = global read "Meas_global.vi" "Analysis Info cluster"() -> (w328:T20[])
        n229 = call "Determine_Meas_Analysis.vi"("Analogue Channels"=w328) -> ("Analysis Info Cluster"=w325:T20[], "Analysis Type Array"=w327:T28[])
        n230 = for {
          tunnel: w325 -> [w338] mode=indexing
          tunnel: w323 -> [w337]
          tunnel: w322 -> [w335]
          tunnel: [w329] -> w321 mode=indexing
          tunnel: [w332] -> w320 mode=indexing
          tunnel: [w331] -> w319 mode=indexing
          i -> [w336]
          w330 = nan ("Mean % Err")
          n231 = Unbundle By Name(w338) -> ("Inst name"=w329:string)
          n232 = Index Array(array=w335, index=w336) -> (element=w334:T27)
          n233 = Index Array(array=w337, index=w336) -> (element=w333:cluster{"Name":string, "Include":bool})
          n234 = Bundle By Name(cluster=w333, "Name"=w329) -> (w332:cluster{"Name":string, "Include":bool})
          n235 = Bundle By Name(cluster=w334, "Name"=w329, "Mean % Err"=w330, "% u'/U"=w330) -> (w331:T27)
        }
        n236 = Build Array (concatenate)("Nothing", w321) -> (w324:string[])
        n237 = local write "Block average display control"(w320) -> ()
        n238 = global write "Meas_global.vi" "Analysis type array"(w327) -> ()
        n239 = global write "Meas_global.vi" "Analysis Info cluster"(w325) -> ()
        n240 = global write "Meas_global.vi" "Velocity Cluster Array"(w319) -> ()
        n241 = property on="Plot 1" class="Ring (strict)"("Strings []"=w324) -> ()  [unwired: 2 in, 2 out]
        n242 = property on="Plot 1" class="Ring (strict)"("Strings []"=w324) -> ()  [unwired: 2 in, 2 out]
        n243 = property on="Plot 2" class="Ring (strict)"("Strings []"=w324) -> ()  [unwired: 2 in, 2 out]
        n244 = property on="Plot 2" class="Ring (strict)"("Strings []"=w324) -> ()  [unwired: 2 in, 2 out]
      }
      frame #11 {
        n245 = global read "Meas_global.vi" "Analysis Info cluster"() -> (w351:T20[])
        n246 = for {
          tunnel: w351 -> [w355] mode=indexing
          tunnel: [w354] -> w350 mode=indexing
          tunnel: [w353] -> w341
          i -> [w353]
          n247 = Unbundle By Name(w355) -> ("Inst name"=w354:string)
        }
        n248 = Greater Than 0?(x=w341) -> (x > 0?=w340:bool)
        n249 = Select(t="Correlate?", s=w340, f=T6."Cross correlation off" ("Correlate?")) -> (s? t:f=w342:T6)
        n250 = global read "Meas_global.vi" "Position"() -> (w349:T7)
        n251 = case shown="\"Correlate without activating panel\"" w342 {
          tunnel: w350 -> [_ w360 w362]
          tunnel: [w357 w359 w361] -> w339
          frame "Cross correlation off" {
            n252 = Initialize Array(0) -> (w357:i32[][])  [unwired: 2 out]
          }
          frame "Show correlation panel" {
            w358 = FALSE  # OK
            n253 = call "Correlation_Display.vi"("Inst names"=w360, "OK"=w358) -> ("correlation array"=w359:i32[][])  [unwired: 2 in, 2 out]
          }
          frame "Correlate without activating panel" {
            n254 = call "Correlation_Display.vi"("Inst names"=w362, "OK"=TRUE) -> ("correlation array"=w361:i32[][])  [unwired: 2 in, 2 out]
          }
        }
        n255 = local write "Position"(w349) -> ()
        n256 = global write "Meas_global.vi" "correlate"(w339) -> ()
        n257 = Array Size(array=w339) -> (size(s)=w348:i32[])
        n258 = Index Array(array=w348, index=0) -> (element=w346:i32)
        n259 = Equal To 0?(x=w346) -> (x = 0?=w345:bool)
        n260 = case shown="True" w345 {
          frame False {
          }
          frame True {
            n261 = local write "Correlate?"(T6."Cross correlation off" ("Correlate?")) -> ()
          }
        }
      }
      frame #12 {
        n262 = stacked-sequence {
          seq-local: [w370 _] -> [_ w392]
          tunnel: w364 -> [w369 _]
          frame #0 {
            n263 = call "LDA+_An_Analysis_mode.vi"("Second Graph"="Second Graph", "First Graph"="First Graph") -> ("Second Graph out"=w365:T3, "First Graph out"=w367:T3)  [unwired: 6 out]
            n264 = case shown="False" w369 {
              tunnel: [w380 w391] -> w368
              tunnel: w367 -> [w379 w391]
              tunnel: [w378 w390] -> w366
              tunnel: w365 -> [w377 w390]
              frame False {
                w375 = Graph_Type."Show no graph" ("Plot Type")
                n265 = Unbundle By Name(w379) -> ("Save graph"=w381:u16)
                n266 = Unbundle By Name(w377) -> ("Save graph"=w376:u16)
                n267 = case shown="0, Default" w381 {
                  tunnel: [w387 w389] -> w380
                  tunnel: w379 -> [w388 w389]
                  tunnel: w375 -> [w386 _]
                  frame 0, Default {
                    n268 = Bundle By Name(cluster=w388, "Plot Type"=w386) -> (w387:T3)
                  }
                  frame 1 {
                  }
                }
                n269 = case shown="0, Default" w376 {
                  tunnel: [w383 w385] -> w378
                  tunnel: w377 -> [w384 w385]
                  tunnel: w375 -> [w382 _]
                  frame 0, Default {
                    n270 = Bundle By Name(cluster=w384, "Plot Type"=w382) -> (w383:T3)
                  }
                  frame 1 {
                  }
                }
              }
              frame True {
              }
            }
            n271 = local write "Second Graph"(w366) -> ()
            n272 = local write "First Graph"(w368) -> ()
            n273 = global write "Meas_global.vi" "Second Graph"(w366) -> ()
            n274 = global write "Meas_global.vi" "First Graph"(w368) -> ()
            n275 = Unbundle By Name(w366) -> ("Plot Type"=w374:T2)
            n276 = Unbundle By Name(w368) -> ("Plot Type"=w373:T2)
            n277 = Build Array(w373, w374) -> (w370:T2[])
          }
          frame #1 {
            n278 = global read "Meas_global.vi" "Insts for plotting"() -> (w393:u16[][])
            n279 = for {
              tunnel: w393 -> [w395] mode=indexing
              tunnel: w392 -> [w394] mode=indexing
              i -> [w396]
              n280 = stacked-sequence {
                seq-local: [w399 _] -> [_ w409]
                seq-local: [w400 _] -> [_ w408]
                tunnel: w396 -> [_ w412]
                tunnel: w395 -> [w398 _]
                tunnel: w394 -> [_ w404]
                frame #0 {
                  n281 = property on="Plot 1" class="Ring (strict)"() -> ("Strings []"=w397:string[])  [unwired: 2 in, 2 out]
                  n282 = Array To Cluster(array=w398) -> (cluster=w403:T30)
                  n283 = Unbundle(w403) -> ("Insts for plotting[0]"=w402:u16, "Insts for plotting[1]"=w401:u16)
                  n284 = Index Array(array=w397, index=w402) -> (element=w399:string)
                  n285 = Index Array(array=w397, index=w401) -> (element=w400:string)
                }
                frame #1 {
                  n286 = case shown="\"Auto-Corr\"" w404 {
                    tunnel: [u8 0 u8 0 u8 0 u8 0 u8 0 u8 1 u8 0] -> w416
                    tunnel: [u8 0 u8 0 u8 0 u8 0 u8 1 u8 1 u8 0] -> w415
                    tunnel: [u8 0 u8 0 u8 0 u8 0 u8 1 u8 1 u8 0] -> w414
                    tunnel: [u8 0 u8 0 u8 0 u8 0 u8 1 u8 0 u8 0] -> w413
                    tunnel: [FALSE TRUE TRUE TRUE TRUE TRUE TRUE] -> w407
                    tunnel: [u8 0 u8 0 u8 0 u8 2 u8 0 u8 0 u8 2] -> w406
                    tunnel: [u8 0 u8 4 u8 1 u8 2 u8 0 u8 0 u8 1] -> w405
                    frame "Show no graph" {
                    }
                    frame "Voltage trace" {
                    }
                    frame "Velocity trace" {
                    }
                    frame "Vel histogram" {
                    }
                    frame "Spectrum" {
                    }
                    frame "f.E(f) v Log f" {
                    }
                    frame "Auto-Corr" {
                    }
                  }
                  n287 = case shown="0, Default" w412 {
                    tunnel: w407 -> [w427 w438]
                    tunnel: w416 -> [w426 w437]
                    tunnel: w415 -> [w425 w436]
                    tunnel: w414 -> [w424 w435]
                    tunnel: w413 -> [w423 w434]
                    tunnel: u32 0 -> [w422 w433]
                    tunnel: u32 1 -> [w421 w431]
                    tunnel: w409 -> [w420 w432]
                    tunnel: w408 -> [w419 w430]
                    tunnel: w406 -> [w418 w429]
                    tunnel: w405 -> [w417 w428]
                    frame 0, Default {
                      n288 = property on="First plot" class="WFGraph (strict)"("Visible"=w427, "X Scale.Format & Precision:Format"=w426, "X Scale.Mapping Mode"=w425, "Y Scale.Format & Precision:Format"=w424, "Y Scale.Mapping Mode"=w423, "Active Plot"=w422, "Plot.Plot Name"=w420, "Active Plot"=w421, "Plot.Plot Name"=w419, "X Scale.Format & Precision:Precision"=w418, "Y Scale.Format & Precision:Precision"=w417) -> ()  [unwired: 2 in, 2 out]
                    }
                    frame 1 {
                      n289 = property on="2nd plot" class="WFGraph (strict)"("Visible"=w438, "X Scale.Format & Precision:Format"=w437, "X Scale.Mapping Mode"=w436, "Y Scale.Format & Precision:Format"=w435, "Y Scale.Mapping Mode"=w434, "Active Plot"=w433, "Plot.Plot Name"=w432, "Active Plot"=w431, "Plot.Plot Name"=w430, "X Scale.Format & Precision:Precision"=w429, "Y Scale.Format & Precision:Precision"=w428) -> ()  [unwired: 2 in, 2 out]
                    }
                  }
                }
              }
            }
          }
        }
      }
      frame #13 {
        n290 = local read "Second Graph"() -> (w499:T3)
        n291 = local read "First Graph"() -> (w498:T3)
        n292 = Unbundle By Name(w498) -> ("Plot 1"=w491:u16, "Plot 2"=w492:u16)
        n293 = Unbundle By Name(w499) -> ("Plot 1"=w493:u16, "Plot 2"=w494:u16)
        n294 = Build Array(w491, w492) -> (w495:u16[])
        n295 = Build Array(w493, w494) -> (w496:u16[])
        n296 = global read "Meas_global.vi" "Analysis Info cluster"() -> (w500:T20[])
        n297 = Decrement(x=w495) -> (x-1=w489:u16[])
        n298 = Decrement(x=w496) -> (x-1=w497:u16[])
        n299 = for {
          tunnel: w500 -> [w508]
          tunnel: w489 -> [w507] mode=indexing
          shift-right: [w501] -> _
          shift-left: u32 0 -> [w503]
          i -> [w502]
          n300 = Index Array(array=w508, index=w507) -> (element=w509:T20)
          n301 = Unbundle By Name(w509) -> ("Colour"=w504:u32)
          n302 = Equal?(x=w504, y=w503) -> (x = y?=w506:bool)
          n303 = Select(t=u32 13434624, s=w506, f=w504) -> (s? t:f=w501:u32)
          n304 = property on="First plot" class="WFGraph (strict)"("Active Plot"=w502, "Plot.Plot Color"=w501, "Plot.Fill/Point Color"=w501) -> ()  [unwired: 2 in, 2 out]
        }
        n305 = for {
          tunnel: w500 -> [w517]
          tunnel: w497 -> [w516] mode=indexing
          shift-right: [w512] -> _
          shift-left: u32 0 -> [w510]
          i -> [w515]
          n306 = Index Array(array=w517, index=w516) -> (element=w518:T20)
          n307 = Unbundle By Name(w518) -> ("Colour"=w511:u32)
          n308 = Equal?(x=w511, y=w510) -> (x = y?=w514:bool)
          n309 = Select(t=u32 13434624, s=w514, f=w511) -> (s? t:f=w512:u32)
          n310 = property on="2nd plot" class="WFGraph (strict)"("Active Plot"=w515, "Plot.Plot Color"=w512, "Plot.Fill/Point Color"=w512) -> ()  [unwired: 2 in, 2 out]
        }
      }
      frame #14 {
        n311 = global read "DataTranslation_global.vi" "Different Sampling Freq per block"() -> (w519:bool)
        n312 = global read "Meas_global.vi" "Remote control"() -> (w528:bool)
        n313 = global read "Meas_global.vi" "Post Process"() -> (w531:T5)
        n314 = global read "Meas_global.vi" "PWA Data"() -> (w520:T31)
        n315 = case shown="\"One Ch PWA\"" w520 {
          tunnel: [w532 w537] -> w522
          frame "No PWA Data" {
            n316 = local read "Desired Sampling freq (Hz)"() -> (w534:dbl)
            n317 = local read "No of samples"() -> (w533:i32)
            n318 = Divide(x=w533, y=w534) -> (x/y=w532:dbl)
          }
          frame "One Ch PWA" {
            n319 = local read "No of samples"() -> (w535:i32)
            n320 = global read "PWAtasksGLOBAL.vi" "PWA Freq. (Hz)"() -> (w536:dbl)
            n321 = global write "PWAtasksGLOBAL.vi" "PWA No. of Samples"(w535) -> ()
            n322 = Divide(x=w535, y=w536) -> (x/y=w537:dbl)
          }
        }
        n323 = global read "Meas_global.vi" "Averaging time (min)"() -> (w526:dbl)
        n324 = Equal?(x=Setup."Run Program" ("setup"), y=w525) -> (x = y?=w523:bool)
        n325 = Equal?(x=Post_Process."Take New Data" ("Post Process"), y=w531) -> (x = y?=w527:bool)
        n326 = Compound Arithmetic op=AND(invert w519, w527, invert w521, invert w528, w523) -> (w529:bool)
        n327 = case shown="True" w529 {
          tunnel: w526 -> [_ w548]
          tunnel: w522 -> [_ w547]
          tunnel: w520 -> [_ w543]
          frame False {
          }
          frame True {
            n328 = global read "Meas_global.vi" "Board type"() -> (w545:T13)
            n329 = Equal?(x=w545, y=Board_Types."Simulate" ("Board type")) -> (x = y?=w539:bool)
            n330 = global read "Meas_global.vi" "LDA data"() -> (w541:enum16{"No LDA data", "Take LDA data"})
            n331 = Equal?(x=enum16{"No LDA data", "Take LDA data"}."Take LDA data" ("LDA data"), y=w541) -> (x = y?=w540:bool)
            n332 = Compound Arithmetic op=AND(invert w540, w539) -> (w538:bool)
            n333 = case shown="False" w538 {
              tunnel: w548 -> [w558 _]
              tunnel: w547 -> [w552 _]
              tunnel: [w551 1 ("No of Blocks")] -> w544
              tunnel: w543 -> [w550 _]
              tunnel: w540 -> [w549 _]
              frame False {
                n334 = Multiply(x=w558, y=60.0) -> (x*y=w556:dbl)
                n335 = Divide(x=w556, y=w552) -> (x/y=w555:dbl)
                n336 = Round Toward +Infinity(x=w555) -> (ceil(x): smallest int >= x=w554:dbl)
                n337 = To Long Integer(number=w554) -> (32bit integer=w553:i32)
                n338 = case shown="\"No PWA Data\"" w550 {
                  tunnel: w549 -> [w562 _]
                  tunnel: w553 -> [w560 w563]
                  tunnel: [w559 w563] -> w551
                  frame "No PWA Data" {
                    n339 = Select(t=99999 ("No of Blocks"), s=w562, f=w560) -> (s? t:f=w559:i32)
                  }
                  frame "One Ch PWA" {
                  }
                }
              }
              frame True {
              }
            }
            n340 = global write "Meas_global.vi" "Requested No of blocks"(w544) -> ()
            n341 = local write "No of Blocks"(w544) -> ()
          }
        }
      }
      frame #15 {
        n342 = case shown="\"Run Program\"" w565 {
          frame "Run Program" {
            n343 = call "Read_calibration_files.vi"() -> ()  [unwired: 1 out]
            n344 = global write "Meas_global.vi" "Repeat Measurement?"(FALSE ("Repeat Measurement?")) -> ()
          }
          frame "Show Setup", Default {
          }
        }
      }
      frame #16 {
        n345 = global read "Meas_global.vi" "Raw data option"() -> (w570:enum16{"Save raw data", "Raw data not saved"})
        n346 = Get Date/Time In Seconds() -> (seconds since 1Jan1904=w571:timestamp)
        n347 = To Double Precision Float(number=w571) -> (double precision float=w568:dbl)
        n348 = global read "Meas_global.vi" "Post Process"() -> (w569:T5)
        n349 = case shown="\"Setup Front Panel\"" w572 {
          tunnel: w570 -> [w575 _ _ _]
          tunnel: w569 -> [w574 _ w607 w616]
          frame "Run Program" {
            n350 = case shown="\"Take New Data\"" w574 {
              tunnel: w575 -> [w576 _]
              frame "Take New Data" {
                n351 = case shown="\"Raw data not saved\"" w576 {
                  frame "Save raw data" {
                  }
                  frame "Raw data not saved" {
                    w584 = FALSE  # Lock File
                    w581 = FALSE  # advisory dialog? (display:T)
                    w580 = FALSE  # append to file? (new file:F)
                    n352 = global read "Meas_global.vi" "Remote control"() -> (w582:bool)
                    n353 = call "Create_setup_string.vi"() -> ("Setup String"=w585:string)  [unwired: 1 out]
                    n354 = case shown="False" w582 {
                      tunnel: ["Current_Setup.xls" ("Setup filename") w587] -> w577
                      frame False {
                      }
                      frame True {
                        n355 = local read "Setup filename"() -> (w587:string)
                      }
                    }
                    n356 = call "Add_length_to_string.vi"("String in"=w585) -> ("String out"=w583:string)
                    n357 = call "Setup_Filepath.vi"("Setup File Type"=Setup_Filetype."Measurement Setups", "Filename in"=w577) -> ("Filename Out"=w578:path)  [unwired: 1 out]
                    n358 = call "Write_Characters_To_File.vi"("file path (dialog if empty)"=w578, "advisory dialog? (display:T)"=w581, "character string"=w583, "append to file? (new file:F)"=w580, "Lock File"=w584) -> ()  [unwired: 4 out]
                  }
                }
              }
              frame "Post Process Raw Data File" {
              }
            }
          }
          frame "Save Current Setup" {
            n359 = stacked-sequence {
              seq-local: [w590 _] -> [_ w593]
              seq-local: [w589 _] -> [_ w592]
              frame #0 {
                w591 = FALSE  # Save New File?
                n360 = call "Save_current_setup.vi"("Save New File?"=w591, "Setup File Type"=Setup_Filetype."Measurement Setups") -> ("Cancelled?"=w589:bool, "Saved filepath"=w590:path)  [unwired: 2 out]
              }
              frame #1 {
                n361 = case shown="False" w592 {
                  tunnel: w593 -> [w599 _]
                  frame False {
                    w596 = "Initial Probe positions" ("File Label")
                    w604 = FALSE  # append to file? (new file:F)
                    w605 = FALSE  # advisory dialog? (display:T)
                    w606 = FALSE  # Lock File
                    n362 = call "Input_Instrument_Positions.vi"("Filepath to Save"=w599) -> ("Output string"=w598:string)  [unwired: 1 out]
                    n363 = call "Create_setup_string.vi"() -> ("Setup String"=w597:string)  [unwired: 1 out]
                    n364 = call "Get_string_subset.vi"("String to split"=w598, "File Label"=w596) -> ("Output string"=w595:string)  [unwired: 2 in, 1 out]
                    n365 = call "Replace_data_in_Label_str.vi"("New data string"=w595, "Input string"=w597, "Variable name"=w596) -> ("Appended string"=w594:string)
                    n366 = call "Replace_data_in_setup_string.vi"("New data string"="", "Input string"=w594, "Variable name"="Comments") -> ("Appended string"=w600:string)
                    n367 = call "Add_length_to_string.vi"("String in"=w600) -> ("String out"=w603:string)
                    n368 = call "Write_Characters_To_File.vi"("file path (dialog if empty)"=w599, "advisory dialog? (display:T)"=w605, "character string"=w603, "append to file? (new file:F)"=w604, "Lock File"=w606) -> ()  [unwired: 4 out]
                  }
                  frame True {
                  }
                }
              }
            }
          }
          frame "Show Setup" {
            n369 = case shown="\"Take New Data\"" w607 {
              frame "Take New Data" {
                w612 = FALSE  # append to file? (new file:F)
                w613 = FALSE  # advisory dialog? (display:T)
                w614 = FALSE  # Lock File
                n370 = call "Create_setup_string.vi"() -> ("Setup String"=w615:string)  [unwired: 1 out]
                n371 = call "Add_length_to_string.vi"("String in"=w615) -> ("String out"=w611:string)
                n372 = call "Setup_Filepath.vi"("Setup File Type"=Setup_Filetype."Measurement Setups", "Filename in"="Current_Setup.xls" ("Setup filename")) -> ("Filename Out"=w609:path)  [unwired: 1 out]
                n373 = call "Write_Characters_To_File.vi"("file path (dialog if empty)"=w609, "advisory dialog? (display:T)"=w613, "character string"=w611, "append to file? (new file:F)"=w612, "Lock File"=w614) -> ()  [unwired: 4 out]
              }
              frame "Post Process Raw Data File" {
              }
            }
          }
          frame "Setup Front Panel" {
            n374 = case shown="\"Take New Data\"" w616 {
              frame "Take New Data" {
                w621 = FALSE  # append to file? (new file:F)
                w622 = FALSE  # advisory dialog? (display:T)
                w623 = FALSE  # Lock File
                n375 = call "Create_setup_string.vi"() -> ("Setup String"=w624:string)  [unwired: 1 out]
                n376 = call "Add_length_to_string.vi"("String in"=w624) -> ("String out"=w620:string)
                n377 = call "Setup_Filepath.vi"("Setup File Type"=Setup_Filetype."Measurement Setups", "Filename in"="Current_Setup.xls" ("Setup filename")) -> ("Filename Out"=w618:path)  [unwired: 1 out]
                n378 = call "Write_Characters_To_File.vi"("file path (dialog if empty)"=w618, "advisory dialog? (display:T)"=w622, "character string"=w620, "append to file? (new file:F)"=w621, "Lock File"=w623) -> ()  [unwired: 4 out]
              }
              frame "Post Process Raw Data File" {
              }
            }
          }
        }
        n379 = call "Program_Active.vi"() -> ()  [unwired: 1 in]
        n380 = global write "Meas_global.vi" "Actual Measurement time (min)"(0.0 ("Max Measurement time (min)")) -> ()
        n381 = global write "Meas_global.vi" "Current Block No"(0 ("Current Block No")) -> ()
      }
      frame #17 {
        n382 = case shown="\"Run Program\"" w628 {
          tunnel: w625 -> [w630 _]
          tunnel: w627 -> [_ w825]
          tunnel: w626 -> [w629 _]
          frame "Run Program" {
            # "LDA2"
            # "PWA"
            # "LDA"
            # "An"
            n383 = stacked-sequence {
              seq-local: [w639 _] -> [_ w663]
              seq-local: [w638 _] -> [_ w662]
              seq-local: [w637 _] -> [_ w661]
              seq-local: [w635 _] -> [_ w660]
              seq-local: [w633 _] -> [_ w657]
              seq-local: [w632 _] -> [_ w656]
              seq-local: [w631 _] -> [_ w655]
              tunnel: w630 -> [_ w659]
              tunnel: w629 -> [_ w658]
              frame #0 {
                n384 = global read "Trav_pos_global.vi" "Dummy Measurement?"() -> (w634:bool)
                n385 = case shown="True" w634 {
                  tunnel: [w647 u16[][] [] ("LDA Binary output")] -> w639
                  tunnel: [w646 w650] -> w638
                  tunnel: [w645 w648] -> w637
                  tunnel: [w644 TRUE ("EOF?")] -> w636
                  tunnel: [w643 T15 {"Started"=0.0, "Ended"=0.0, "Analogue Frequency Hz"=1000.0} ("Block Timings")] -> w635
                  tunnel: [w642 w650] -> w633
                  tunnel: [w641 ""] -> w632
                  tunnel: [w640 w648] -> w631
                  frame False {
                    n386 = call "Get_data.vi"() -> ("EOF? and Error status"=w644:bool, "Voltage output"=w645:dbl[][], "Analogue Binary"=w646:i16[][], "LDA Binary output"=w647:u16[][], "Block Timings"=w643:T15, "PWA Binary"=w642:i16[][], "Block Header"=w641:string, "LDA 2nd Group"=w640:dbl[][])  [unwired: 4 out]
                  }
                  frame True {
                    w648 = dbl[][] [] ("Voltage output")
                    w650 = i16[][] [] ("Analogue Binary")
                  }
                }
                n387 = case shown="True" w636 {
                  frame False {
                  }
                  frame True {
                    n388 = local write "No of Blocks"(1 ("No of Blocks")) -> ()
                  }
                }
              }
              frame #1 {
                n389 = while {
                  tunnel: w659 -> [w671]
                  shift-left: w660 -> [w672]
                  shift-right: [w673] -> _
                  shift-left: w661 -> [w677]
                  shift-right: [w680] -> _
                  shift-left: w662 -> [w678]
                  shift-right: [w681] -> _
                  shift-left: w663 -> [w679]
                  shift-right: [w682] -> _
                  tunnel: w658 -> [w670]
                  shift-right: [w669] -> _
                  shift-left: w657 -> [w668]
                  shift-right: [w667] -> _
                  shift-left: w656 -> [w666]
                  shift-right: [w665] -> _
                  shift-left: w655 -> [w664]
                  i -> [w674]
                  stop <- w683 continue-if-true
                  n390 = Increment(x=w674) -> (x+1=w684:i32)
                  n391 = stacked-sequence {
                    seq-local: [w686 _ _] -> [_ w697 _]
                    seq-local: [_ w696 _] -> [_ _ w718]
                    tunnel: [_ w700 _] -> w682
                    tunnel: [_ w699 _] -> w681
                    tunnel: [_ w698 _] -> w680
                    tunnel: "No of Blocks" -> [w691 _ _]
                    tunnel: "stop" -> [w689 _ _]
                    tunnel: w674 -> [w687 _ w717]
                    tunnel: [_ w695 _] -> w673
                    tunnel: [_ w694 _] -> w669
                    tunnel: [_ w693 _] -> w667
                    tunnel: [_ w692 _] -> w665
                    frame #0 {
                      n392 = Increment(x=w687) -> (x+1=w685:i32)
                      "Current Block No" <- w685
                      n393 = Less Or Equal?(x=w691, y=w685) -> (x <= y?=w690:bool)
                      n394 = Or(x=w690, y=w689) -> (x .or. y?=w688:bool)
                      n395 = Not(x=w688) -> (.not. x?=w686:bool)
                      n396 = global write "Meas_global.vi" "Current Block No"(w685) -> ()
                    }
                    frame #1 {
                      n397 = case shown="False" w697 {
                        tunnel: [u16[][] [] ("LDA Binary output") w714] -> w700
                        tunnel: [w703 w713] -> w699
                        tunnel: [w701 w712] -> w698
                        tunnel: [FALSE ("EOF?") w711] -> w696
                        tunnel: [T15 {"Started"=0.0, "Ended"=0.0, "Analogue Frequency Hz"=200.0} ("Block Timings") w710] -> w695
                        tunnel: [w703 w709] -> w694
                        tunnel: ["" w708] -> w693
                        tunnel: [w701 w707] -> w692
                        frame False {
                          w701 = dbl[][] [] ("Voltage output")
                          w703 = i16[][] [] ("Analogue Binary")
                        }
                        frame True {
                          n398 = call "Get_data.vi"() -> ("EOF? and Error status"=w711:bool, "Voltage output"=w712:dbl[][], "Analogue Binary"=w713:i16[][], "LDA Binary output"=w714:u16[][], "Block Timings"=w710:T15, "PWA Binary"=w709:i16[][], "Block Header"=w708:string, "LDA 2nd Group"=w707:dbl[][])  [unwired: 4 out]
                        }
                      }
                    }
                    frame #2 {
                      n399 = Increment(x=w717) -> (x+1=w715:i32)
                      n400 = Increment(x=w715) -> (x+1=w716:i32)
                      n401 = case shown="True" w718 {
                        tunnel: w716 -> [_ w719]
                        frame False {
                        }
                        frame True {
                          n402 = local write "No of Blocks"(w719) -> ()
                        }
                      }
                    }
                  }
                  n403 = stacked-sequence {
                    seq-local: [_ _ _ _ _ "Block average display control" _ _ _ _] -> [_ _ _ _ _ _ w782 _ _ _]
                    seq-local: [_ _ _ _ _ _ w779 _ _ _] -> [_ _ _ _ _ _ _ w793 _ _]
                    seq-local: [w723 _ _ _ _ _ _ _ _ _] -> [_ w729 _ _ w765 _ _ _ _ w823]
                    seq-local: [_ _ w734 _ _ _ _ _ _ _] -> [_ _ _ _ w763 _ _ _ _ _]
                    seq-local: [_ _ _ w755 _ _ _ _ _ _] -> [_ _ _ _ w764 _ _ _ _ _]
                    tunnel: w684 -> [w722 _ _ _ w767 w775 _ _ _ _]
                    tunnel: [_ _ _ _ _ _ _ _ _ w823] -> w683
                    tunnel: w674 -> [_ _ _ _ _ _ _ _ _ _]
                    tunnel: w679 -> [_ _ _ w753 _ _ _ _ _ _]
                    tunnel: w678 -> [_ _ _ w752 _ _ _ _ _ _]
                    tunnel: w677 -> [_ _ _ w759 _ _ _ _ _ _]
                    tunnel: "stop" -> [w725 _ _ _ _ _ _ _ _ _]
                    tunnel: "No of Blocks" -> [w724 _ _ _ _ _ _ _ _ _]
                    tunnel: w672 -> [_ _ _ w757 _ _ _ _ _ _]
                    tunnel: w671 -> [_ _ w733 w754 _ _ _ _ _ _]
                    tunnel: w670 -> [_ _ w735 _ _ _ _ _ _ _]
                    tunnel: w668 -> [_ _ _ w751 _ _ _ _ _ _]
                    tunnel: w666 -> [w721 _ _ _ _ _ _ _ _ _]
                    tunnel: w664 -> [w720 _ _ _ _ _ _ _ _ _]
                    frame #0 {
                      n404 = global write "Plug_in_data_global.vi" "Block Header"(w721) -> ()
                      n405 = global write "LDA_meas_global_2.vi" "LDA 2nd Group"(w720) -> ()
                      n406 = Less Or Equal?(x=w724, y=w722) -> (x <= y?=w727:bool)
                      n407 = Or(x=w725, y=w727) -> (x .or. y?=w726:bool)
                      n408 = global write "Meas_global.vi" "Current Block No"(w722) -> ()
                      n409 = Not(x=w726) -> (.not. x?=w723:bool)
                    }
                    frame #1 {
                      n410 = call "Program_Active.vi"() -> ()  [unwired: 1 in]
                      n411 = call "Text_without_format.vi"("Input string"="Comments") -> ("Output string"=w730:string)
                      n412 = global write "Meas_global.vi" "Position"("Position") -> ()
                      n413 = local write "Comments"(w730) -> ()
                      n414 = global write "Meas_global.vi" "Comments"(w730) -> ()
                      n415 = Not(x=w729) -> (.not. x?=w728:bool)
                      n416 = global write "Meas_global.vi" "Processing last block?"(w728) -> ()
                      n417 = global write "PWAtasksGLOBAL.vi" "STOP"(w728) -> ()
                    }
                    frame #2 {
                      n418 = case shown="False" w733 {
                        tunnel: w735 -> [w747 _]
                        tunnel: [w736 FALSE] -> w734
                        frame False {
                          w744 = 1.5  # To allow for overhead
                          n419 = Get Date/Time In Seconds() -> (seconds since 1Jan1904=w749:timestamp)
                          n420 = global read "Meas_global.vi" "Averaging time (min)"() -> (w743:dbl)
                          n421 = To Double Precision Float(number=w749) -> (double precision float=w748:dbl)
                          n422 = Subtract(x=w748, y=w747) -> (x-y=w746:dbl)
                          n423 = global read "Meas_global.vi" "LDA data"() -> (w740:enum16{"No LDA data", "Take LDA data"})
                          n424 = Divide(x=w746, y=60.0 ("To convert to minutes")) -> (x/y=w742:dbl)
                          n425 = Equal?(x=enum16{"No LDA data", "Take LDA data"}."Take LDA data" ("LDA data"), y=w740) -> (x = y?=w737:bool)
                          n426 = Multiply(x=w744, y=w743) -> (x*y=w741:dbl)
                          n427 = Greater?(x=w742, y=w741) -> (0:w738:bool)
                          n428 = And(x=w737, y=w738) -> (x .and. y?=w736:bool)
                        }
                        frame True {
                        }
                      }
                    }
                    frame #3 {
                      n429 = call "Process_data.vi"("PWA Binary"=w751, "Analogue Binary"=w752, "LDA Binary output"=w753, "Analogue volts"=w759, "Measurement top level?"=w754, "Block Timings"=w757) -> ("Vel stat display"=→"Statistics":string[][], "First Plot data"=→"First plot":cluster{"Xo":dbl, "Delta X":dbl, dbl[]}[], "Second Plot data"=→"2nd plot":cluster{"Xo":dbl, "Delta X":dbl, dbl[]}[], "Max Measurement time up"=w755:bool)
                    }
                    frame #4 {
                      n430 = global read "Meas_global.vi" "stop"() -> (w762:bool)
                      n431 = Compound Arithmetic op=OR(w762, w763, w764) -> (w761:bool)
                      n432 = And(x=w765, y=w761) -> (x .and. y?=w766:bool)
                      n433 = case shown="True" w766 {
                        tunnel: w767 -> [_ w768]
                        frame False {
                        }
                        frame True {
                          n434 = Increment(x=w768) -> (x+1=w769:i32)
                          n435 = local write "No of Blocks"(w769) -> ()
                        }
                      }
                    }
                    frame #5 {
                      n436 = global read "Meas_global.vi" "Actual Measurement time (min)"() -> (→"Measurement time (min)":dbl)
                      n437 = global read "Meas_global.vi" "Actual Sampling rate (Hz)"() -> (→"Actual Sampling freq":dbl)
                      n438 = call "Display_blocks.vi"("Block No"=w775, "Block average display"="Block average display control") -> ("u^4"=→"u^4":dbl[][], "u^3"=→"u^3":dbl[][], "uv"=→"uv":dbl[][], "u^2"=→"u^2" →"Array u^2":dbl[][], "U"=→"U" →"Array U":dbl[][])  [unwired: 4 out]
                    }
                    frame #6 {
                      n439 = global read "Meas_global.vi" "Analysis Info cluster"() -> (w781:T20[])
                      n440 = for {
                        tunnel: w782 -> [w787] mode=indexing
                        shift-right: [w783] -> w779
                        shift-left: u32[] [] -> [w784]
                        tunnel: w781 -> [w786] mode=indexing
                        n441 = Unbundle By Name(w787) -> ("Include"=w785:bool)
                        n442 = case shown="True" w785 {
                          tunnel: w786 -> [_ w792]
                          tunnel: w784 -> [w788 w790]
                          tunnel: [w788 w789] -> w783
                          frame False {
                          }
                          frame True {
                            n443 = Unbundle By Name(w792) -> ("Colour"=w791:u32)
                            n444 = Build Array (concatenate)(w790, w791) -> (w789:u32[])
                          }
                        }
                      }
                    }
                    frame #7 {
                      n445 = for {
                        tunnel: w793 -> [w794] mode=indexing
                        i -> [w795]
                        n446 = property on="U" class="WFGraph (strict)"("Active Plot"=w795, "Plot.Plot Color"=w794, "Plot.Fill/Point Color"=w794) -> ()  [unwired: 2 in, 2 out]
                        n447 = property on="u^3" class="WFGraph (strict)"("Active Plot"=w795, "Plot.Plot Color"=w794, "Plot.Fill/Point Color"=w794) -> ()  [unwired: 2 in, 2 out]
                        n448 = property on="u^4" class="WFGraph (strict)"("Active Plot"=w795, "Plot.Plot Color"=w794, "Plot.Fill/Point Color"=w794) -> ()  [unwired: 2 in, 2 out]
                        n449 = property on="u^2" class="WFGraph (strict)"("Active Plot"=w795, "Plot.Plot Color"=w794, "Plot.Fill/Point Color"=w794) -> ()  [unwired: 2 in, 2 out]
                      }
                    }
                    frame #8 {
                      n450 = case shown="True" "Pause" {
                        frame False {
                        }
                        frame True {
                          n451 = global read "Meas_global.vi" "Post Process"() -> (w797:T5)
                          n452 = case shown="\"Take New Data\"" w797 {
                            frame "Take New Data" {
                              n453 = call "Program_Active_Client.vi"("Mode"=enum16{"Program Active", "Traverse Level State"}."Program Active", "Time till next contact (Sec)"=12000.0, "Traverse level State"=Traverse_Level_State."Running") -> ()  [unwired: 3 out]
                              n454 = while {
                                i -> [w804]
                                stop <- w805 continue-if-true
                                n455 = Quotient & Remainder(x=w804, y=10) -> (x-y*floor(x/y)=w802:i32)  [unwired: 1 out]
                                n456 = Equal To 0?(x=w802) -> (x = 0?=w801:bool)
                                n457 = stacked-sequence {
                                seq-local: [_ w807 _ _] -> [_ _ w809 _]
                                tunnel: [_ w807 _ _] -> w805
                                tunnel: w801 -> [_ _ _ w811]
                                frame #0 {
                                "Pause message" <- "Measurement Program Paused!!!!" ("Pause message")
                                }
                                frame #1 {
                                n458 = global write "Trav_pos_global.vi" "Paused During Row?"(TRUE ("Paused During Row?")) -> ()
                                n459 = local read "Pause"() -> (w807:bool)
                                }
                                frame #2 {
                                n460 = property on="Pause message" class="Str"("Blinking"=w809, "Visible"=w809) -> ()  [unwired: 2 in, 2 out]
                                n461 = Wait Until Next ms Multiple(millisecond multiple=u32 1000) -> ()  [unwired: 1 out]
                                }
                                frame #3 {
                                n462 = case shown="False" w811 {
                                frame False {
                                }
                                frame True {
                                n463 = Current VI's Path() -> (path=w812:path)
                                n464 = call "Bring_to_front.vi"("path"=w812) -> ()
                                }
                                }
                                }
                                }
                              }
                            }
                            frame "Post Process Raw Data File" {
                              n465 = stacked-sequence {
                                seq-local: [_ w815 _ _] -> [_ _ _ w822]
                                frame #0 {
                                n466 = property on="PP next block" class="Bool (strict)"("Visible"=TRUE) -> ()  [unwired: 2 in, 2 out]
                                n467 = local write "PP next block"(FALSE ("PP next block")) -> ()
                                }
                                frame #1 {
                                n468 = while {
                                tunnel: [w819] -> w815
                                stop <- w816 stop-if-true
                                n469 = local read "stop"() -> (w819:bool)
                                n470 = local read "Pause"() -> (w817:bool)
                                n471 = Compound Arithmetic op=OR(w819, "PP next block", invert w817) -> (w816:bool)
                                n472 = case shown="False" w816 {
                                frame False {
                                n473 = Wait (ms)(milliseconds to wait=u32 200) -> ()  [unwired: 1 out]
                                }
                                frame True {
                                }
                                }
                                }
                                }
                                frame #2 {
                                n474 = property on="PP next block" class="Bool (strict)"("Visible"=FALSE) -> ()  [unwired: 2 in, 2 out]
                                }
                                frame #3 {
                                n475 = Stop(stop? (T)=w822) -> ()
                                }
                              }
                            }
                          }
                        }
                      }
                    }
                    frame #9 {
                      n476 = global read "Meas_global.vi" "Diagnostic info"() -> (→"BSA Diagnostic info":string[][])
                    }
                  }
                }
              }
            }
          }
          frame "Setup Front Panel", Default {
            n477 = stacked-sequence {
              seq-local: [w826 _ _ _ _ _ _] -> [_ _ _ _ _ w900 _]
              seq-local: [_ w832 _ _ _ _ _] -> [_ _ _ _ _ w899 _]
              seq-local: [_ _ _ w863 _ _ _] -> [_ _ _ _ _ w898 _]
              seq-local: [_ _ _ _ w876 _ _] -> [_ _ _ _ _ w896 _]
              seq-local: [_ w831 _ _ _ _ _] -> [_ _ _ _ _ _ w913]
              seq-local: [_ _ w857 _ _ _ _] -> [_ _ _ _ _ w895 _]
              tunnel: w825 -> [_ w833 _ _ _ _ _]
              frame #0 {
                n478 = Build Array("Name", "Channel", "High limit", "Low limit") -> (w826:string[])
              }
              frame #1 {
                n479 = global read "Meas_global.vi" "LDA data"() -> (w831:enum16{"No LDA data", "Take LDA data"})
                n480 = case shown="\"Take LDA data\"" w831 {
                  tunnel: w833 -> [_ w844]
                  tunnel: [string[][] [] w841] -> w832
                  frame "No LDA data" {
                  }
                  frame "Take LDA data" {
                    n481 = global read "LDA_meas_global_1.vi" "Max Vel BSA1"() -> (w836:dbl)
                    n482 = global read "LDA_meas_global_1.vi" "Vel Comp BSA1"() -> (w845:string)
                    n483 = global read "LDA_meas_global_1.vi" "Min Vel BSA1"() -> (w835:dbl)
                    n484 = case shown="\"2D\"" w844 {
                      tunnel: [string[] [] w850] -> w842
                      frame "1D" {
                      }
                      frame "2D" {
                        n485 = global read "LDA_meas_global_2.vi" "Max Vel BSA2"() -> (w849:dbl)
                        n486 = global read "LDA_meas_global_2.vi" "Min Vel BSA2"() -> (w848:dbl)
                        n487 = global read "LDA_meas_global_2.vi" "Vel Comp BSA2"() -> (w851:string)
                        n488 = Format Into String(format string="%.1f m/s" ("Format String"), w848) -> (resulting string=w856:string)  [unwired: 2 in, 1 out]
                        n489 = Format Into String(format string="%.1f m/s" ("Format String"), w849) -> (resulting string=w855:string)  [unwired: 2 in, 1 out]
                        n490 = Build Array("LDA", w851, w855, w856) -> (w850:string[])
                      }
                    }
                    n491 = Format Into String(format string="%.1f m/s" ("Format String"), w835) -> (resulting string=w837:string)  [unwired: 2 in, 1 out]
                    n492 = Format Into String(format string="%.1f m/s" ("Format String"), w836) -> (resulting string=w838:string)  [unwired: 2 in, 1 out]
                    n493 = Build Array("LDA", w845, w838, w837) -> (w843:string[])
                    n494 = Build Array(w843, w842) -> (w841:string[][])
                  }
                }
              }
              frame #2 {
                n495 = global read "Meas_global.vi" "PWA Data"() -> (w858:T31)
                n496 = case shown="\"One Ch PWA\"" w858 {
                  tunnel: [string[][] [] w860] -> w857
                  frame "No PWA Data" {
                  }
                  frame "One Ch PWA" {
                    n497 = Build Array("PWA") -> (w861:string[])
                    n498 = Build Array(w861) -> (w860:string[][])
                  }
                }
              }
              frame #3 {
                n499 = global read "Meas_global.vi" "Ch & spans"() -> (w864:T26[])
                n500 = for {
                  tunnel: w864 -> [w875] mode=indexing
                  tunnel: [w871] -> w863 mode=indexing
                  n501 = Unbundle By Name(w875) -> ("Var name"=w874:string, "Ch No"=w873:i16, "high limit (10V)"=w868:sgl, "low limit (-10V)"=w867:sgl)
                  n502 = Format Into String(format string="%.1f Volts" ("Format String"), w868) -> (resulting string=w866:string)  [unwired: 2 in, 1 out]
                  n503 = Format Into String(format string="%.1f Volts" ("Format String"), w867) -> (resulting string=w865:string)  [unwired: 2 in, 1 out]
                  n504 = Number To Decimal String(number=w873) -> (decimal integer string=w872:string)  [unwired: 1 out]
                  n505 = Build Array(w874, w872, w866, w865) -> (w871:string[])
                }
              }
              frame #4 {
                n506 = global read "Meas_global.vi" "Analysis Info cluster"() -> (w884:T20[])
                n507 = for {
                  tunnel: w884 -> [w894] mode=indexing
                  tunnel: [w893] -> w882 mode=indexing
                  n508 = Unbundle By Name(w894) -> ("Inst name"=w893:string)
                }
                n509 = global read "Meas_global.vi" "correlate"() -> (w883:i32[][])
                n510 = for {
                  tunnel: w883 -> [w889] mode=indexing
                  tunnel: w882 -> [w888]
                  tunnel: "Correlating" -> [w887]
                  tunnel: [w885] -> w877 mode=indexing
                  n511 = for {
                    tunnel: w889 -> [w892] mode=indexing
                    tunnel: w888 -> [w891]
                    tunnel: [w890] -> w886 mode=indexing
                    n512 = Index Array(array=w891, index=w892) -> (element=w890:string)
                  }
                  n513 = Build Array (concatenate)(w887, w886) -> (w885:string[])
                }
                n514 = Initialize Array("", 5 ("Dimension Size")) -> (w878:string[])
                n515 = Build Array (concatenate)(w878, w877) -> (w876:string[][])
              }
              frame #5 {
                n516 = Build Array (concatenate)(w900, w899, w895, w898, w896) -> (w897:string[][])
                n517 = local write "Statistics"(w897) -> ()
              }
              frame #6 {
                n518 = global read "Meas_global.vi" "Board type"() -> (w911:T13)
                n519 = global read "Meas_global.vi" "Continuous time trace?"() -> (w912:bool)
                n520 = Equal?(x=w911, y=Board_Types."ADC488" ("Board type")) -> (x = y?=w909:bool)
                n521 = case shown="\"Take LDA data\"" w913 {
                  tunnel: w909 -> [_ w917]
                  tunnel: [string[] [] w916] -> w905
                  frame "No LDA data" {
                  }
                  frame "Take LDA data" {
                    n522 = global read "Meas_global.vi" "Synchronise with LDA"() -> (w922:bool)
                    n523 = global read "Meas_global.vi" "Ch & spans"() -> (w925:T26[])
                    n524 = global read "LDA_meas_global_1.vi" "Probe Configuration"() -> (w915:string)
                    n525 = Array Size(array=w925) -> (size(s)=w924:i32)
                    n526 = Greater Than 0?(x=w924) -> (x > 0?=w923:bool)
                    n527 = Compound Arithmetic op=AND(w922, w917, w923) -> (w921:bool)
                    n528 = Select(t="Synchronised with LDA", s=w921, f="") -> (s? t:f=w918:string)
                    n529 = Build Array(w915, w918) -> (w916:string[])
                  }
                }
                n530 = Compound Arithmetic op=AND(w909, w912) -> (w906:bool)
                n531 = Select(t="Continuous Time Trace", s=w906, f="") -> (s? t:f=w904:string)
                n532 = Build Array (concatenate)(w905, w904) -> (w903:string[])
                n533 = Build Array(w903) -> (w902:string[][])
                n534 = Transpose 2D Array(2D array=w902) -> (transposed array=w901:string[][])
                n535 = local write "BSA Diagnostic info"(w901) -> ()
              }
            }
          }
        }
      }
      frame #18 {
        n536 = local read "File"() -> (w943:T9)
        n537 = Equal?(x=Setup."Run Program" ("setup"), y=w944) -> (x = y?=w941:bool)
        n538 = Not Equal?(x=w943, y=Save_Data."Save No Data" ("File")) -> (x != y?=w942:bool)
        n539 = global read "Meas_global.vi" "Repeat Measurement?"() -> (w926:bool)
        n540 = Compound Arithmetic op=AND(invert w926, w941, w942) -> (w940:bool)
        n541 = Get Date/Time In Seconds() -> (seconds since 1Jan1904=w937:timestamp)
        n542 = To Double Precision Float(number=w937) -> (double precision float=w929:dbl)
        n543 = local read "Setup filename"() -> (w938:string)
        n544 = global read "Trav_pos_global.vi" "Meas Setup Number"() -> (w935:i32)
        n545 = global read "Meas_global.vi" "Board type"() -> (w933:T13)
        n546 = Greater Than 0?(x=w935) -> (x > 0?=w931:bool)
        n547 = Equal?(x=w933, y=Board_Types."Simulate" ("Board type")) -> (x = y?=w932:bool)
        n548 = And(x=w931, y=w932) -> (x .and. y?=w930:bool)
        n549 = case shown="True" w930 {
          tunnel: w929 -> [_ w948]
          tunnel: [w945 w946] -> w928
          tunnel: w927 -> [w945 _]
          frame False {
          }
          frame True {
            n550 = global read "Trav_pos_global.vi" "Current Row"() -> (w951:T17)
            n551 = Unbundle By Name(w951) -> ("Averaging time (min)"=w949:dbl)
            n552 = Multiply(x=60.0 ("y"), y=w949) -> (x*y=w947:dbl)
            n553 = Subtract(x=w948, y=w947) -> (x-y=w946:dbl)
          }
        }
        n554 = case shown="True" w940 {
          tunnel: w943 -> [_ _]
          tunnel: w929 -> [w954 w1006]
          tunnel: w938 -> [w953 w1005]
          tunnel: w928 -> [w952 w1004]
          frame True {
            n555 = stacked-sequence {
              seq-local: [_ w958 _ _ _] -> [_ _ w964 _ _]
              seq-local: [_ _ _ w977 _] -> [_ _ _ _ w997]
              tunnel: w954 -> [w957 _ _ _ _]
              tunnel: w953 -> [w956 _ _ _ _]
              tunnel: w952 -> [w955 _ _ _ _]
              frame #0 {
                n556 = call "Write_Results_file.vi"("Experiment start time"=w955, "Experiment End time"=w957, "Setup filename"=w956) -> ()  [unwired: 4 out]
              }
              frame #1 {
                n557 = global read "Meas_global.vi" "Second Graph"() -> (w962:T3)
                n558 = global read "Meas_global.vi" "First Graph"() -> (w963:T3)
                n559 = Unbundle By Name(w962) -> ("Save graph"=w960:u16)
                n560 = Unbundle By Name(w963) -> ("Save graph"=w961:u16)
                n561 = Add(x=w961, y=w960) -> (x+y=w959:u16)
                n562 = Not Equal To 0?(x=w959) -> (x != 0?=w958:bool)
              }
              frame #2 {
                n563 = case shown="True" w964 {
                  frame False {
                  }
                  frame True {
                    n564 = stacked-sequence {
                      tunnel: "Show Smoth" -> [w968 w969]
                      frame #0 {
                        n565 = local read "First plot"() -> (w967:cluster{"Xo":dbl, "Delta X":dbl, dbl[]}[])
                        n566 = local read "2nd plot"() -> (w966:cluster{"Xo":dbl, "Delta X":dbl, dbl[]}[])
                        n567 = call "Save_plot_routine.vi"("Show Smooth"=w968, "First Plot data"=w967, "Second Plot data"=w966) -> ()  [unwired: 1 in, 3 out]
                      }
                      frame #1 {
                        n568 = case shown="True" w969 {
                          frame False {
                          }
                          frame True {
                            n569 = Open VI Reference(vi path="Measurement.vi") -> (vi reference=w975:refnum<vi>, error out=w971:errorcluster)  [unwired: 1 in, 4 out]
                            n570 = local write "Show Smoth"(FALSE ("Show Smoth")) -> ()
                            n571 = property class="VI"(reference=w975, error in=w971, "Front Panel Window:Is Frontmost"=TRUE) -> (reference out=w973:refnum<vi>, error out=w972:errorcluster)
                            n572 = Close Reference(reference=w973, error in (no error)=w972) -> ()  [unwired: 1 out]
                          }
                        }
                      }
                    }
                  }
                }
              }
              frame #3 {
                w982 = FALSE  # Empty list
                n573 = global read "Meas_global.vi" "Raw data file"() -> (w981:path)
                n574 = global read "Trav_pos_global.vi" "Top level setup filename"() -> (w979:path)
                n575 = global read "Meas_global.vi" "Start Time of experiment"() -> (w978:dbl)
                n576 = Strip Path(path=w981) -> (stripped path=w977:path)  [unwired: 1 out]
                n577 = Empty String/Path?(string/path=w979) -> (empty?=w980:bool)
                n578 = case shown="False" w980 {
                  tunnel: w979 -> [w996 _]
                  tunnel: w977 -> [w994 _]
                  tunnel: w978 -> [w992 _]
                  frame False {
                    n579 = call "Sec_to_date_filename.vi"("seconds"=w992) -> ("Day"=w991:string, "Time"=w990:string)  [unwired: 2 out]
                    n580 = Format Into String(format string="Cmd_%s_%s.xls", w991, w990) -> (resulting string=w988:string)  [unwired: 2 in, 1 out]
                    n581 = call "Fast_string_Replace.vi"("Replace match with:"="-", "Input String"=w988, "regular expression"=":") -> ("Output String"=w985:string)  [unwired: 2 out]
                    n582 = call "Fast_string_Replace.vi"("Replace match with:"="", "Input String"=w985, "regular expression"=" ") -> ("Output String"=w983:string)  [unwired: 2 out]
                    n583 = Build Path(base path=w994, name or relative path=w983) -> (appended path=w993:path)
                    n584 = Copy(10:w993, 11:w996) -> ()  [unwired: 1 in, 5 out]
                  }
                  frame True {
                  }
                }
                n585 = call "Remember_RD_Folders.vi"("Empty list"=w982, "Folders to Remember"=w977) -> ()  [unwired: 1 out]
              }
              frame #4 {
                n586 = global read "Meas_global.vi" "LDA data"() -> (w998:enum16{"No LDA data", "Take LDA data"})
                n587 = case shown="\"Take LDA data\"" w998 {
                  tunnel: w997 -> [_ w1002]
                  frame "No LDA data" {
                  }
                  frame "Take LDA data" {
                    w1000 = "LDA_Probe_Orientation.txt" ("name or relative path")
                    n588 = call "Setup_Filepath.vi"("Setup File Type"=Setup_Filetype."General", "Filename in"=w1000) -> ("Filename Out"=w999:path)  [unwired: 1 out]
                    n589 = Build Path(base path=w1002, name or relative path=w1000) -> (appended path=w1003:path)
                    n590 = Copy(10:w1003, 11:w999) -> ()  [unwired: 1 in, 5 out]
                  }
                }
              }
            }
          }
          frame False {
            n591 = global read "Meas_global.vi" "Raw data option"() -> (w1007:enum16{"Save raw data", "Raw data not saved"})
            n592 = case shown="\"Save raw data\"" w1007 {
              tunnel: w1004 -> [w1010 _]
              tunnel: w1006 -> [w1009 _]
              tunnel: w1005 -> [w1008 _]
              frame "Save raw data" {
                n593 = stacked-sequence {
                  tunnel: w1010 -> [_ w1019]
                  tunnel: w1009 -> [_ w1018]
                  tunnel: w1008 -> [_ w1016]
                  frame #0 {
                    n594 = global read "Meas_global.vi" "Current Block No"() -> (w1011:i32)
                    n595 = global write "Meas_global.vi" "Requested No of blocks"(w1011) -> ()
                  }
                  frame #1 {
                    n596 = call "Create_Raw_data_file.vi"("No of averages"=1, "End time"=w1018, "Start time"=w1019, "Setup filename"=w1016) -> ("Values"=w1014:string[][], "Column headers"=w1015:string[])  [unwired: 2 out]
                    n597 = Index Array(array=w1014, index (row)=0) -> (element=w1012:string[])  [unwired: 1 in]
                    n598 = global write "Dynamic_call_global.ph.vi" "Plug in values"(w1012) -> ()
                    n599 = global write "Dynamic_call_global.ph.vi" "Plug in titles"(w1015) -> ()
                  }
                }
              }
              frame "Raw data not saved" {
              }
            }
          }
        }
      }
      frame #19 {
        n600 = stacked-sequence {
          seq-local: [w1026 _] -> [_ w1035]
          seq-local: [w1022 _] -> [_ w1034]
          tunnel: w1020 -> [w1033 _]
          frame #0 {
            n601 = global read "Meas_global.vi" "Raw data file"() -> (w1024:path)
            n602 = global read "Meas_global.vi" "Raw data option"() -> (w1032:enum16{"Save raw data", "Raw data not saved"})
            n603 = Equal?(x=Setup."Run Program" ("setup"), y=w1033) -> (x = y?=w1028:bool)
            n604 = Strip Path(path=w1024) -> (stripped path=w1023:path)  [unwired: 1 out]
            n605 = Equal?(x=w1032, y=enum16{"Save raw data", "Raw data not saved"}."Save raw data" ("Raw data option")) -> (x = y?=w1027:bool)
            n606 = Build Path(base path=w1023, name or relative path="VI_History.xls") -> (appended path=w1022:path)
            n607 = call "Does_file_exist_(simple).vi"("Pathname"=w1022) -> ("exists?"=w1030:bool)
            n608 = Not(x=w1030) -> (.not. x?=w1029:bool)
            n609 = Compound Arithmetic op=AND(w1029, w1028, w1027) -> (w1026:bool)
          }
          frame #1 {
            n610 = case shown="True" w1035 {
              tunnel: w1034 -> [_ w1041]
              frame False {
              }
              frame True {
                w1038 = FALSE  # Lock File
                n611 = global read "Meas_global.vi" "ProgRevisionInfo"() -> (w1037:string)
                n612 = call "Characters_to_string.vi"("Characters to write"=w1037, "Label for characters"="Prog Revision info") -> ("Output string"=w1043:string)
                n613 = call "Date_and_Time_to_string.vi"() -> ("Date and time (spreadsheet)"=w1044:string)
                n614 = call "Get_mod_dates.vi"() -> ("error out"=w1042:errorcluster, "Output string"=w1039:string)  [unwired: 1 in, 3 out]
                n615 = call "EnFlo_Error_Handler.vi"("error in (no error)"=w1042) -> ()  [unwired: 2 in, 3 out]
                n616 = Concatenate Strings(w1044, w1043, w1039) -> (w1040:string)
                n617 = call "Write_Characters_To_File.vi"("file path (dialog if empty)"=w1041, "character string"=w1040, "Lock File"=w1038) -> ()  [unwired: 2 in, 4 out]
              }
            }
          }
        }
      }
      frame #20 {
        w1047 = FALSE ("Remote control")
        n618 = local read "Correlate?"() -> (w1049:T6)
        n619 = case shown="\"Run Program\"" w1046 {
          tunnel: w1046 -> [w1053 _ _ _]
          tunnel: [w1053 w1070 w1071 w1072] -> w1045
          frame "Run Program" {
            n620 = global read "Meas_global.vi" "Velocity Cluster Array"() -> (w1052:T27[])
            n621 = Array Size(array=w1052) -> (size(s)=w1051:i32)
            n622 = Decrement(x=w1051) -> (x-1=w1050:i32)
            n623 = while {
              tunnel: w1052 -> [w1068] mode=indexing
              tunnel: w1050 -> [w1059]
              i -> [w1060]
              stop <- w1057 continue-if-true
              w1065 = "Pitot ("
              n624 = Unbundle By Name(w1068) -> ("U"=w1054:dbl, "Name"=w1064:string)
              n625 = String Length(string=w1065) -> (length=w1067:i32)
              n626 = String Subset(string=w1064, length (rest)=w1067) -> (substring=w1066:string)  [unwired: 1 out]
              n627 = Equal?(x=w1066, y=w1065) -> (x = y?=w1061:bool)
              n628 = call "Match_Pat_Case_In.vi"("String to match"="ref", "String"=w1064) -> ("offset past match"=w1062:i32)  [unwired: 1 in, 3 out]
              n629 = Greater Or Equal To 0?(x=w1062) -> (x >= 0?=w1056:bool)
              n630 = Less?(x=w1060, y=w1059) -> (x < y?=w1058:bool)
              n631 = And(x=w1056, y=w1061) -> (x .and. y?=w1055:bool)
              n632 = case shown="True" w1055 {
                tunnel: w1054 -> [_ w1069]
                frame False {
                }
                frame True {
                  n633 = call "Log_Reference_Velocity.vi"("Measured Velocity"=w1069) -> ()  [unwired: 1 out]
                }
              }
              n634 = Compound Arithmetic op=AND(invert w1055, w1058) -> (w1057:bool)
            }
          }
          frame "Show Setup" {
            w1070 = Setup."Run Program"  # setup
          }
          frame "Save Current Setup" {
            w1071 = Setup."Run Program"  # setup
          }
          frame "Setup Front Panel" {
            w1072 = Setup."Run Program"  # setup
          }
        }
        n635 = case shown="\"Correlate without activating panel\"" w1049 {
          tunnel: [T6."Cross correlation off" T6."Correlate without activating panel" T6."Correlate without activating panel"] -> w1048
          frame "Cross correlation off" {
          }
          frame "Show correlation panel" {
          }
          frame "Correlate without activating panel" {
          }
        }
        n636 = local write "Correlate?"(w1048) -> ()
        n637 = global write "Meas_global.vi" "Remote control"(w1047) -> ()
        n638 = global write "Dynamic_call_global.ph.vi" "Acquisition Interlock"(w1047) -> ()
        n639 = call "Program_Active.vi"() -> ()  [unwired: 1 in]
        n640 = local write "setup"(w1045) -> ()
      }
      frame #21 {
        w1080 = FALSE  # Dialog Box (T)
        n641 = global read "Meas_global.vi" "Over/Under string"() -> (w1078:string)
        n642 = Empty String/Path?(string/path=w1078) -> (empty?=w1077:bool)
        n643 = Not(x=w1077) -> (.not. x?=w1076:bool)
        n644 = Bundle By Name(cluster=errorcluster {"status"=FALSE, "code"=0, "source"=""} ("error in (no error)"), "source"=w1078, "status"=w1076) -> (w1081:errorcluster)
        n645 = call "EnFlo_Error_Handler.vi"("error in (no error)"=w1081, "Error Type"="Signal Clipping", "Dialog Box (T)"=w1080) -> ()  [unwired: 3 out]
      }
      frame #22 {
        w1085 = string[] [] ("Per Block Plug Ins Extra")
        n646 = Empty String/Path?(string/path=w1089) -> (empty?=w1088:bool)
        n647 = global read "Dynamic_call_global.ph.vi" "Final Plug Ins"() -> (w1090:string[])
        n648 = case shown="True" w1088 {
          tunnel: w1089 -> [w1102 _]
          frame False {
            n649 = local read "Comments"() -> (w1101:string)
            n650 = call "Fast_string_Replace.vi"("Replace match with:"="", "Input String"=w1101, "regular expression"=w1102) -> ("Output String"=w1100:string)  [unwired: 2 out]
            n651 = local write "Comments"(w1100) -> ()
          }
          frame True {
          }
        }
        n652 = call "Plug_in_Directories.vi"() -> ("Final"=w1086:path)  [unwired: 3 out]
        n653 = for {
          tunnel: w1090 -> [w1105] mode=indexing
          tunnel: w1086 -> [w1104]
          w1108 = FALSE  # Dialog Box (T)
          n654 = Build Path(base path=w1104, name or relative path=w1105) -> (appended path=w1103:path)
          n655 = global read "Dynamic_call_global.ph.vi" "Plug in"() -> (w1113:refnum<vi>)
          n656 = Open VI Reference(type specifier VI Refnum (for type only)=w1113, vi path=w1103) -> (vi reference=w1112:refnum<vi>, error out=w1111:errorcluster)  [unwired: 2 in, 2 out]
          n657 = call-by-ref "?"(reference=w1112, error in=w1111) -> (reference out=w1109:refnum<vi>, error out=w1110:errorcluster)  [unwired: 6 in, 2 out]
          n658 = Close Reference(reference=w1109, error in (no error)=w1110) -> (error out=w1106:errorcluster)
          n659 = call "EnFlo_Error_Handler.vi"("error in (no error)"=w1106, "Error Type"="Running Final Plug In", "Dialog Box (T)"=w1108) -> ()  [unwired: 3 out]
        }
        n660 = global read "Meas_global.vi" "Repeat Measurement?"() -> (w1087:bool)
        n661 = case shown="False" w1087 {
          tunnel: w1084 -> [_ w1098]
          tunnel: [FALSE w1093] -> w1083
          frame False {
            n662 = global write "Trav_pos_global.vi" "Present Probe Positions"(T7 [] ("Present Probe Positions")) -> ()
          }
          frame True {
            n663 = global read "Meas_global.vi" "Post Process"() -> (w1096:T5)
            n664 = Equal To 0?(x=w1098) -> (x = 0?=w1094:bool)
            n665 = Equal?(x=w1096, y=Post_Process."Post Process Raw Data File" ("Post Process")) -> (x = y?=w1095:bool)
            n666 = And(x=w1095, y=w1094) -> (x .and. y?=w1093:bool)
          }
        }
        n667 = global write "Dynamic_call_global.ph.vi" "Per Block Plug Ins Extra"(w1085) -> ()
        n668 = global write "Dynamic_call_global.ph.vi" "Initial Plug Ins Extra"(w1085) -> ()
      }
      frame #23 {
        n669 = global read "Meas_global.vi" "Post Process"() -> (w1120:T5)
        n670 = local read "stop"() -> (w1126:bool)
        n671 = Equal?(x=w1121, y=Setup."Run Program" ("setup")) -> (x = y?=w1117:bool)
        n672 = Equal?(x=w1120, y=Post_Process."Take New Data" ("Post Process")) -> (x = y?=w1118:bool)
        n673 = And(x=w1117, y=w1118) -> (x .and. y?=w1116:bool)
        n674 = case shown="False" w1126 {
          tunnel: [Multi_Run_Status."Continue" ("Status Out") Multi_Run_Status."Terminate Run" ("Status Out")] -> w1124
          frame False {
          }
          frame True {
            n675 = local write "stop"(FALSE) -> ()
          }
        }
        n676 = case shown="True" w1116 {
          tunnel: w1124 -> [w1127 w1130]
          tunnel: [w1127 w1132] -> w1123
          frame False {
          }
          frame True {
            n677 = local read "Raw data file"() -> (w1131:path)
            n678 = Path to Array of Strings(0:w1131) -> (2:w1133:string[])  [unwired: 1 out]
            n679 = Index Array(array=w1133, index=0 ("Index")) -> (element=w1129:string)
            n680 = Build Array(w1129) -> (w1128:string[])
            n681 = for {
              tunnel: w1128 -> [w1137] mode=indexing
              shift-right: [w1135] -> w1132
              shift-left: w1130 -> [w1136]
              n682 = call "Warn_on_low_HD_space.vi"("Status In"=w1136, "HD name"=w1137) -> ("Status Out"=w1135:T4)  [unwired: 6 out]
            }
          }
        }
        "Status Out" <- w1123
        n683 = global write "Trav_pos_global.vi" "Dummy Measurement?"(FALSE ("Dummy Measurement?")) -> ()
        n684 = global write "Plug_in_data_global.vi" "Server Channels to log"(string[] [] ("Server Channels to log")) -> ()
        n685 = global write "Meas_global.vi" "Extra Comments"("") -> ()
      }
    }
  }
